vi "GyroServoControl.vi"() -> ()   [LabVIEW 2017]
uses:
  MsgTypeDef.ctl
  <vilib>/WPC Systems Ltd/GECO Driver/Lib/GECOMotion/GECOMotion/_typedefine/Axis Select.ctl
  <vilib>/WPC Systems Ltd/GECO Driver/Lib/GECOMotion/GECOMotion/GECO Motion.lvclass
  <vilib>/WPC Systems Ltd/GECO Driver/Lib/GECOBase/GECO_Driver Class/Motion/_typedefine/GECO_Motion Operation Mode.ctl
  <vilib>/WPC Systems Ltd/GECO Driver/Lib/GECOBase/GECO_Driver Class/GECO_Driver.lvclass
  <vilib>/WPC Systems Ltd/GECO Driver/Lib/GECOBase/GECO_Driver Class/Motion/_typedefine/GECO_ActiveHighLow.ctl
  <vilib>/addons/control/pid/NI_PID_pid.lvlib
  <vilib>/addons/control/pid/pid.llb/PID (DBL).vi
  <vilib>/NI/Modbus Library/API/Wrapper/API Main.lvlib
  GyroDef.ctl
  DataDef.ctl
  <vilib>/WPC Systems Ltd/GECO Driver/Lib/GECOBase/GECO_Driver Class/GECO_SlotName.ctl
  <vilib>/WPC Systems Ltd/GECO Driver/Lib/GECOBase/GECO_Driver Class/Motion/_typedefine/GECO_Stepper Output Configuration.ctl
  <vilib>/NI/Modbus Library/API/Modbus API.lvclass
  <vilib>/Instr/_visa.llb/VISA Configure Serial Port (Instr).vi
  <vilib>/NI/Modbus Library/API/Wrapper/Create TCP Slave.vi
  <vilib>/WPC Systems Ltd/GECO Driver/GECODriver/GECO_Initialize_PC/Initialize VIs/Initialize_GECOUno_4HX.vi
  <vilib>/NI/Modbus Library/API/Slave/Modbus Slave.lvclass
  C:/Program Files (x86)/National Instruments/LabVIEW 2019/vi.lib/NI/Modbus Library/API/Modbus API.lvclass
  Motion Controller Slot.ctl
  Reverse Polarity.ctl
  Forward Polarity.ctl
  Stepper Output Configuration.ctl
  Axis Select.ctl
panel:
  out "error IO 2":errorcluster
  out "error IO":errorcluster
  out "Gyro\nPeriod":u32
  out "Program Period":u32
  out "Axis 3":T1
  out "Axis 2":T1
  out "Axis 1":T1
  in  "ServoButtonControl":T2
  in  "Main Setting Tab":T3(tab)
  in  "TimerON":bool
  in  "Timer(ms)":i32=1
  in  "Serial Port":refnum<visa-resource-name>="COM3"
  in  "TCP slave port":u32=1
  in  "baud rate":u32=115200
  in  "Byte bits":u32=8
  in  "Modbus Address Starting":u32
  in  "Modbus Number of Inputs":u32=10000
  in  "Resource Name":tag="rio://192.168.0.224/RIO0"
  in  "Servo on":bool
  in  "Axis Select":T4
  in  "Stepper Output Configuration":T5=enum."CW/CCW(Two Pulse)"
  in  "Forward Enable?":bool=TRUE
  in  "Reverse Enable?":bool=TRUE
  in  "Motion Operation Mode":T6(ring)=enum."Velocity"
  in  "Forward Polarity":T7
  in  "Reverse Polarity":T8
  in  "Motion Controller Slot":T9
  in  "Target Position (0)":dbl=10000.0
  in  "Acceleration (100000)":u32=300000
  in  "Velocity (10000)":dbl=100000.0
  in  "Deacceleration (100000)":u32=300000
  in  "PID gains setting Tab":enum32{"Axis 1", "Axis 2", "Axis 3"}(tab)
  in  "PID gains":T10={"proportional gain (Kc)"=0.75, "integral time (Ti, min)"=0.01, "derivative time (Td, min)"=0.0} {"derivative time (Td, min)" format="%#_3f"; "integral time (Ti, min)" format="%#_3f"; "proportional gain (Kc)" format="%#_3f"}
  in  "PID gains 2":T10={"proportional gain (Kc)"=0.75, "integral time (Ti, min)"=0.01, "derivative time (Td, min)"=0.0} {"derivative time (Td, min)" format="%#_3f"; "integral time (Ti, min)" format="%#_3f"; "proportional gain (Kc)" format="%#_3f"}
  in  "PID gains 3":T10={"proportional gain (Kc)"=0.75, "integral time (Ti, min)"=0.01, "derivative time (Td, min)"=0.0} {"derivative time (Td, min)" format="%#_3f"; "integral time (Ti, min)" format="%#_3f"; "proportional gain (Kc)" format="%#_3f"}
  in  "ZABStop":bool
  in  "B":i32
  in  "A":i32
  in  "Z":i32=50
  in  "ZAB Start":bool
  in  "Move Setting":T11
  in  "Close":bool
  in  "Connect":bool
  out "實際角度":cluster{"A":dbl, "B":dbl}={"A"=-3.299667554384925, "B"=3.520332445615068}
  out "register values":dbl[](array[numeric])
  out "實際角度Chart":cluster{"X":dbl, "Y":dbl}(graph)={"X"=-3.299667554384925, "Y"=3.520332445615068} caption="Waveform Chart - dark"
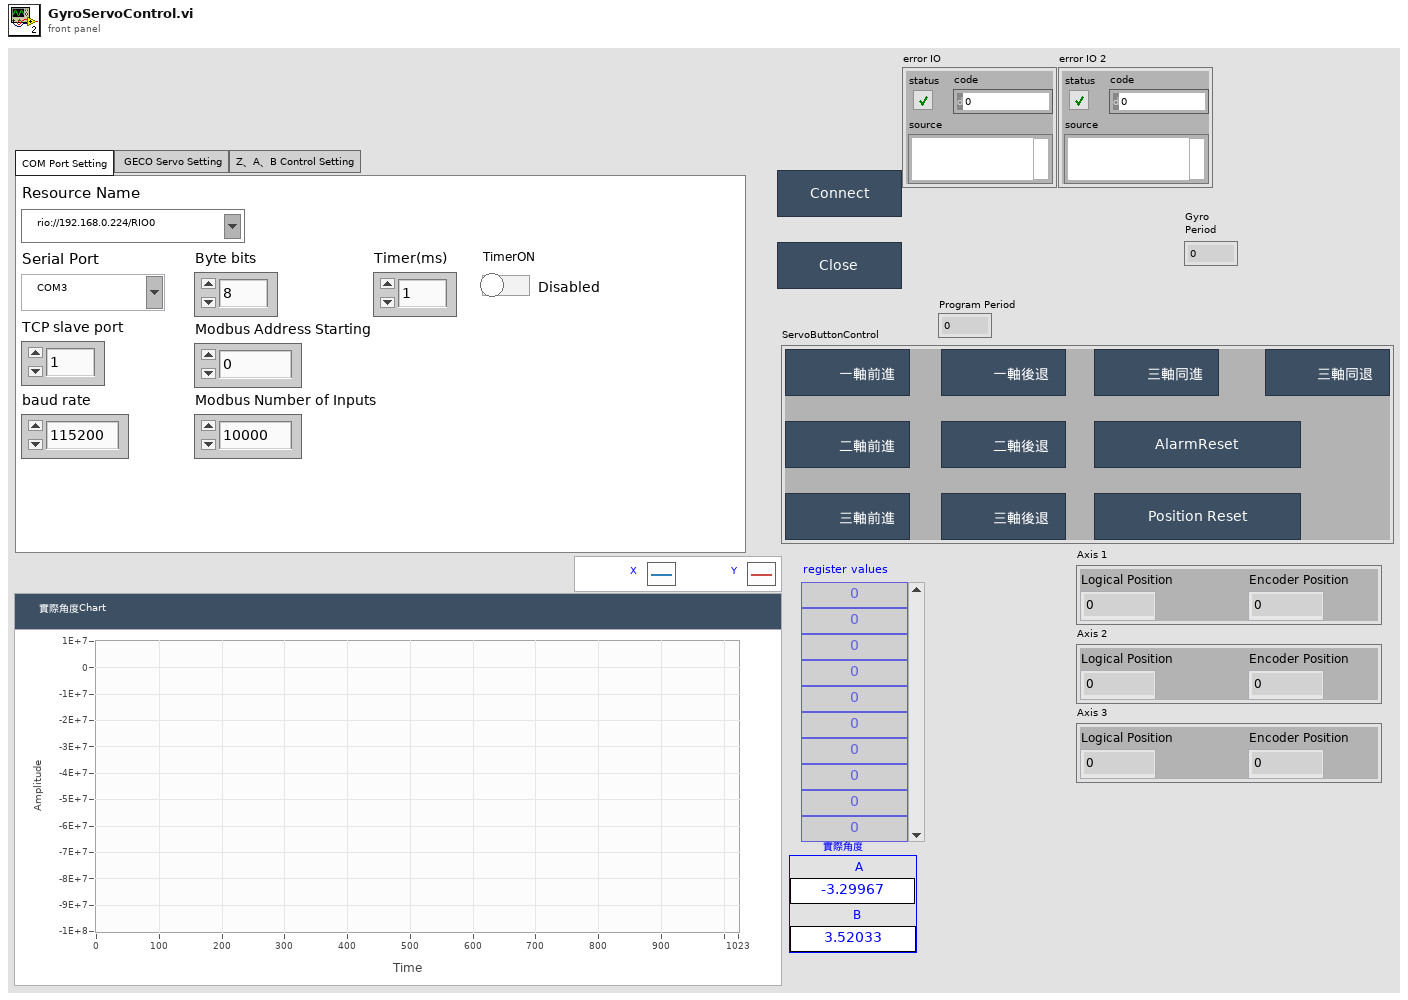
[diagram p1: front panel]
types:
  T1 = cluster{"Encoder Position":i32, "Logical Position":i32}
  T2 = cluster{"三軸同退":bool, "三軸同進":bool, "三軸後退":bool, "三軸前進":bool, "二軸後退":bool, "二軸前進":bool, "一軸後退":bool, "一軸前進":bool, "Reset Encoder Position":bool, "AlarmReset":bool}
  T3 = enum32{"COM Port Setting", " GECO Servo Setting", "Z、A、B Control Setting"}
  T4 = typedef "Axis Select.ctl" = enum16{"Axis 1", "Axis 2", "Axis 3", "Axis 4"}
  T5 = typedef "Stepper Output Configuration.ctl" = enum16{"Step/Dir(One Pulse)", "CW/CCW(Two Pulse)"}
  T6 = enum16{"Absolute Position", "Relative Position", "Velocity"}
  T7 = typedef "Forward Polarity.ctl" = enum16{"Active High", "Active Low"}
  T8 = typedef "Reverse Polarity.ctl" = enum16{"Active High", "Active Low"}
  T9 = typedef "Motion Controller Slot.ctl" = enum16{"C1", "C2", "C3", "C4"}
  T10 = cluster{"proportional gain (Kc)":dbl, "integral time (Ti, min)":dbl, "derivative time (Td, min)":dbl}
  T11 = typedef "軌跡設定.ctl" = u16
  T12 = typedef "MsgTypeDef.ctl" = cluster{"CMD":string, "DATA":variant}
  T13 = typedef "GyroDef.ctl" = cluster{"Byte bits":u16, "baud rate":u32, "實際角度":cluster{"A":dbl, "B":dbl}, "COM Port":refnum<visa-resource-name>, "Save Path":refnum<file>}
  T14 = typedef "DataDef.ctl" = cluster{"address starting":u16, "狀態":enum16{"初始化", "讀取", "寫入", "停止"}, "理想角度":cluster{"A":dbl, "B":dbl}, "register values":i16[], "Modbus COM":refnum<class "Modbus API.lvclass">, "TCP slave port":u16, " baud rate":u32, "Byte bits":u16, "ServoButtonControl":cluster{"三軸同退":bool, "三軸同進":bool, "三軸後退":bool, "三軸前進":bool, "二軸後退":bool, "二軸前進":bool, "一軸後退":bool, "一軸前進":bool}, "Serial Number":string, "GECO_Driver out":refnum<class "GECO_Driver.lvclass">, "number of inputs":u16, "ServoSetting":cluster{"Axis Select":T15, "Stepper Output Configuration":T16, "Motion Operation Mode":T17, "Motion Controller Slot":T18, "Singel Axis Move Paramters":cluster{"Motion Operation Mode":T17, "Target Position (0)":i32, "Velocity (10000)":i32, "Acceleration (100000)":u32, "Deacceleration (100000)":u32}, "Reverse":cluster{"Reverse Enable":bool, "Reverse Polarity":T19}, "Forward":cluster{"Forward Enable":bool, "Forward Polarity":T19}}, "GECO Motion out":refnum<class "GECO Motion.lvclass">, "Servo on":bool, "Axis 1 Position":cluster{"Encoder Position":i32, "Logical Position":i32}, "Axis 2 Position":cluster{"Encoder Position":i32, "Logical Position":i32}, "Axis 3 Position":cluster{"Encoder Position":i32, "Logical Position":i32}, "PIDSetting":cluster{"Z":i32, "A":i32, "B":i32, "Move Setting":T20, "Axis Pulse":dbl, "Axis Length":dbl, "PID gains ":cluster{"proportional gain (Kc)":dbl, "integral time (Ti, min)":dbl, "derivative time (Td, min)":dbl}}, "resource name":tag, "Save Path":refnum<file>}
  T15 = typedef "GECO Motion.lvclass/Axis Select.ctl" = enum16{"Axis 1", "Axis 2", "Axis 3", "Axis 4"}
  T16 = typedef "GECO_Driver.lvclass/GECO_Stepper Output Configuration.ctl" = enum16{"Step/Dir(One Pulse)", "CW/CCW(Two Pulse)"}
  T17 = typedef "GECO_Driver.lvclass/GECO_Motion Operation Mode.ctl" = enum16{"Absolute Position", "Relative Position", "Velocity"}
  T18 = typedef "GECO_Driver.lvclass/GECO_SlotName.ctl" = enum16{"C1", "C2", "C3", "C4"}
  T19 = typedef "GECO_Driver.lvclass/GECO_ActiveHighLow.ctl" = enum16{"Active High", "Active Low"}
  T20 = typedef "­y¸ñ.ctl" = u16
  T21 = cluster{"Motion Operation Mode":T17, "Target Position (0)":i32, "Velocity (10000)":i32, "Acceleration (100000)":u32, "Deacceleration (100000)":u32}
  T22 = cluster{"Forward Enable":bool, "Forward Polarity":T19}
  T23 = cluster{"Reverse Enable":bool, "Reverse Polarity":T19}
  T24 = cluster{"三軸同退":bool, "三軸同進":bool, "三軸後退":bool, "三軸前進":bool, "二軸後退":bool, "二軸前進":bool, "一軸後退":bool, "一軸前進":bool, "Reset Encoder Position":bool, "AlarmReset":bool}[]
  T25 = enum16{"open", "replace", "create", "open or create", "replace or create", "replace or create with confirmation"}
  T26 = cluster{"Logical Position":i32, "Encoder Position":i32}
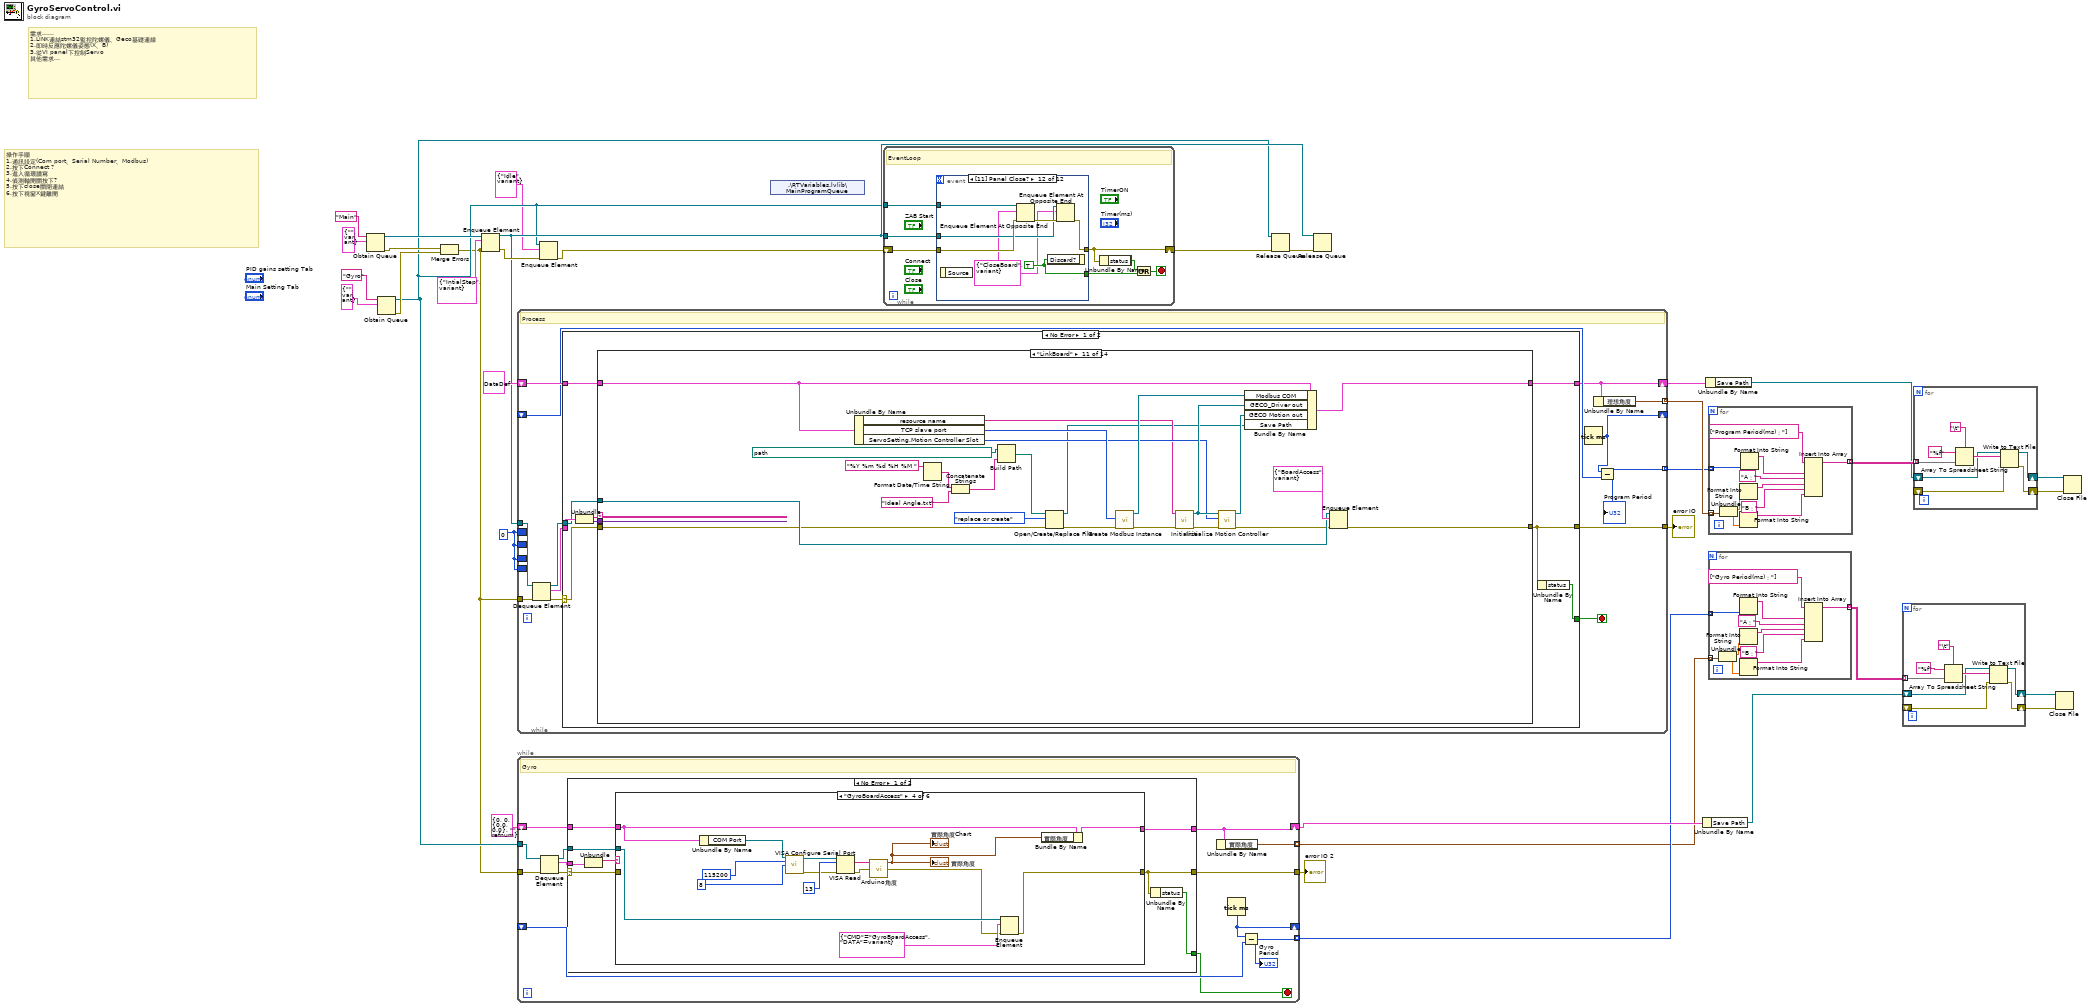
[diagram p0: block diagram]
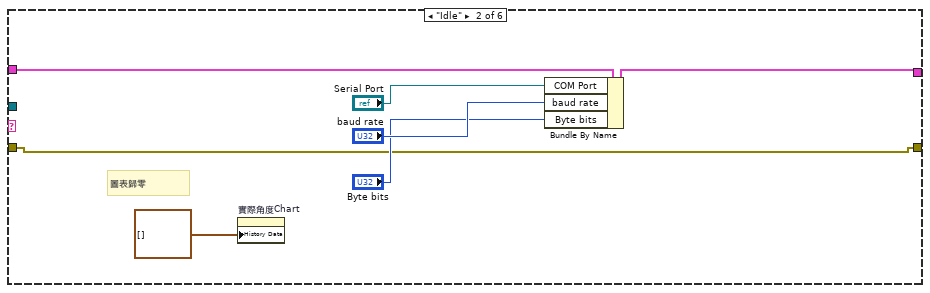
[diagram p3: hidden frame]
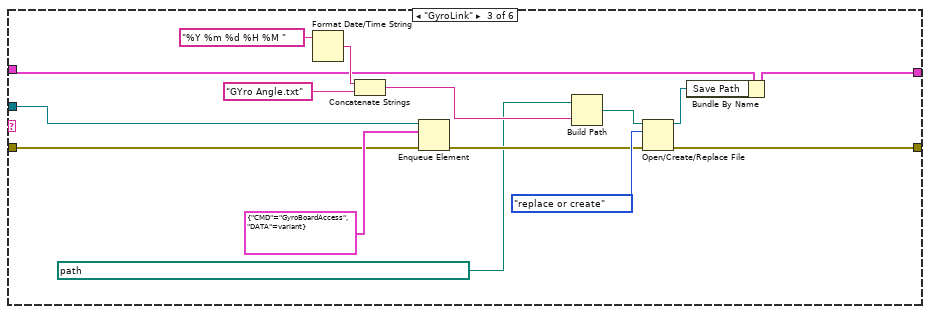
[diagram p4: hidden frame]
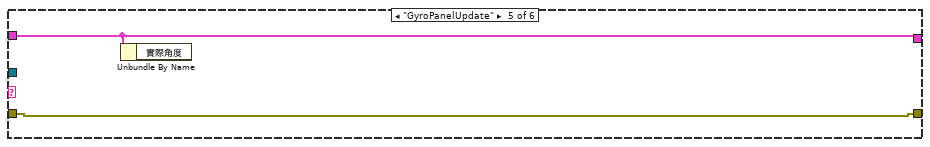
[diagram p5: hidden frame]
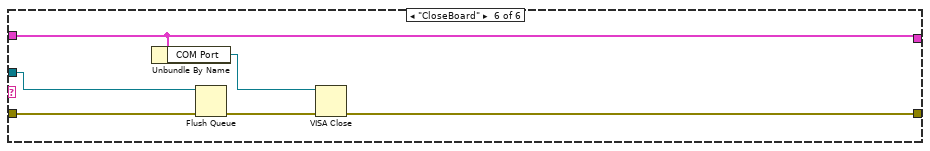
[diagram p6: hidden frame]
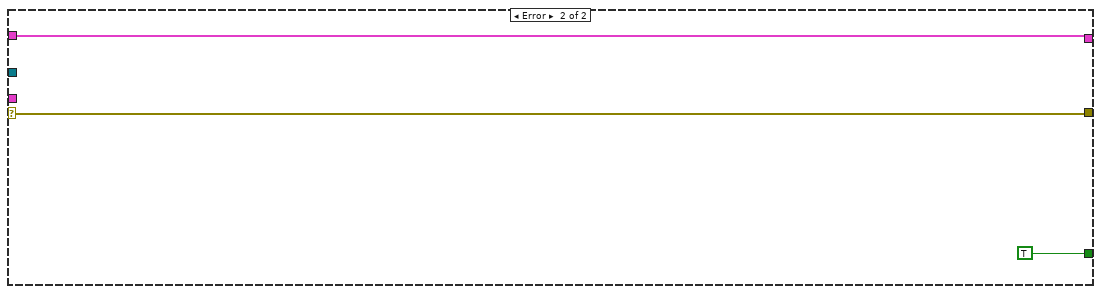
[diagram p7: hidden frame]
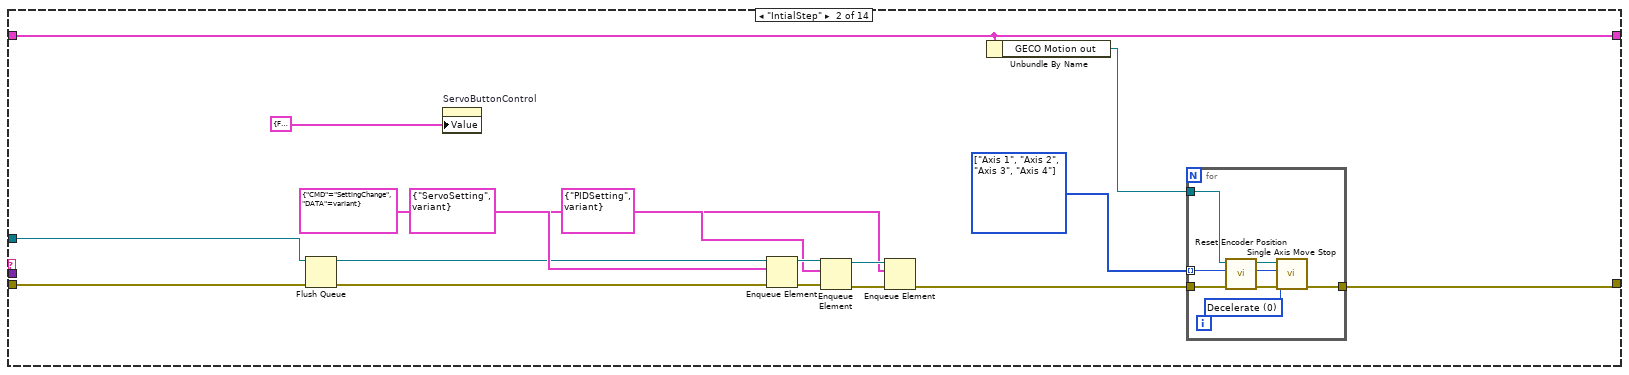
[diagram p9: hidden frame]
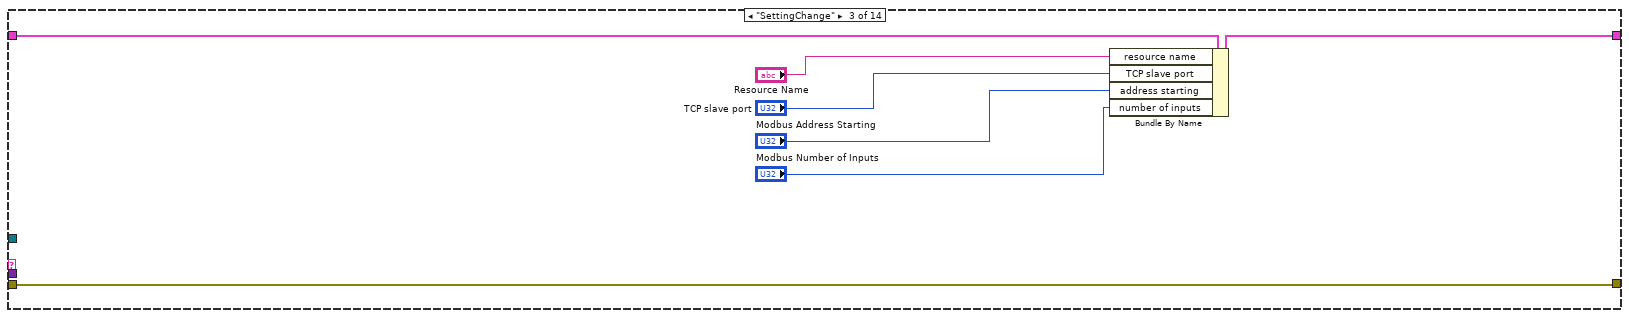
[diagram p10: hidden frame]
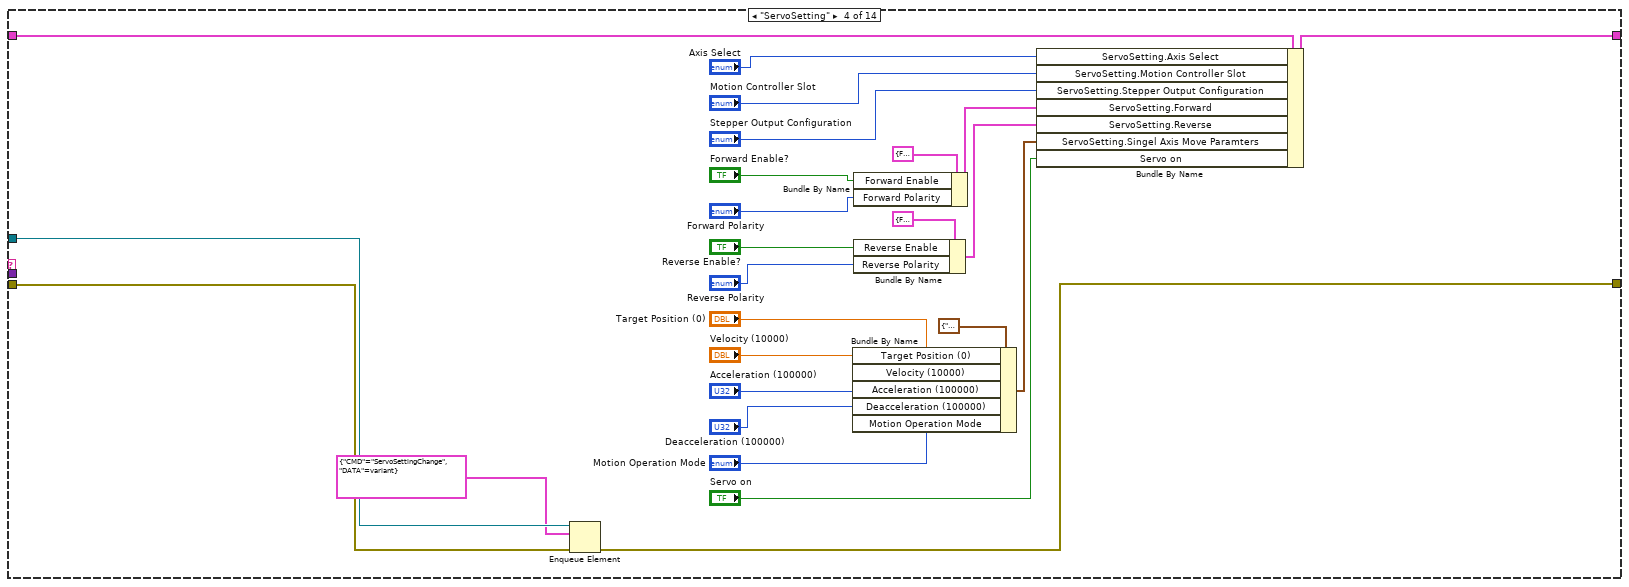
[diagram p11: hidden frame]
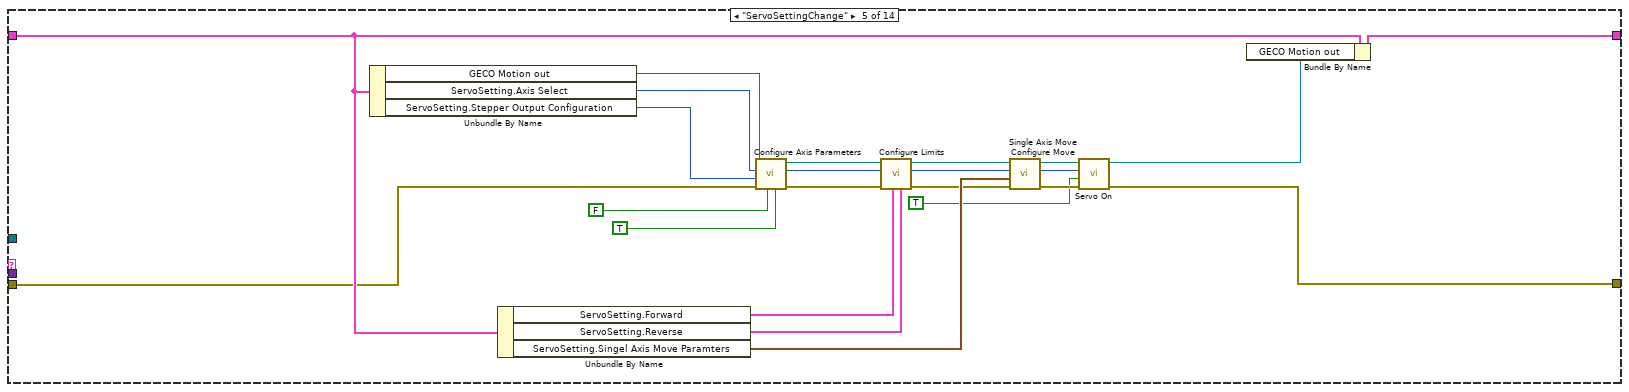
[diagram p12: hidden frame]
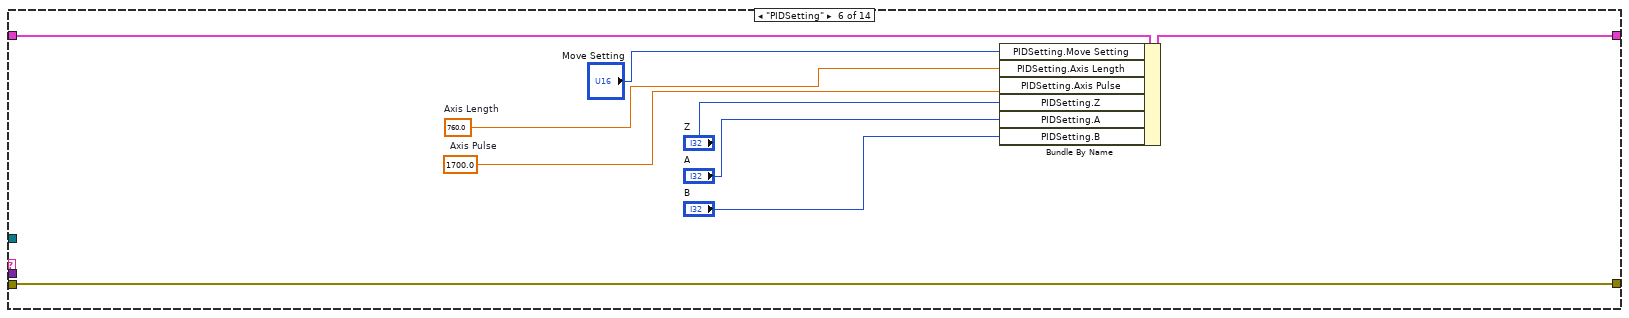
[diagram p13: hidden frame]
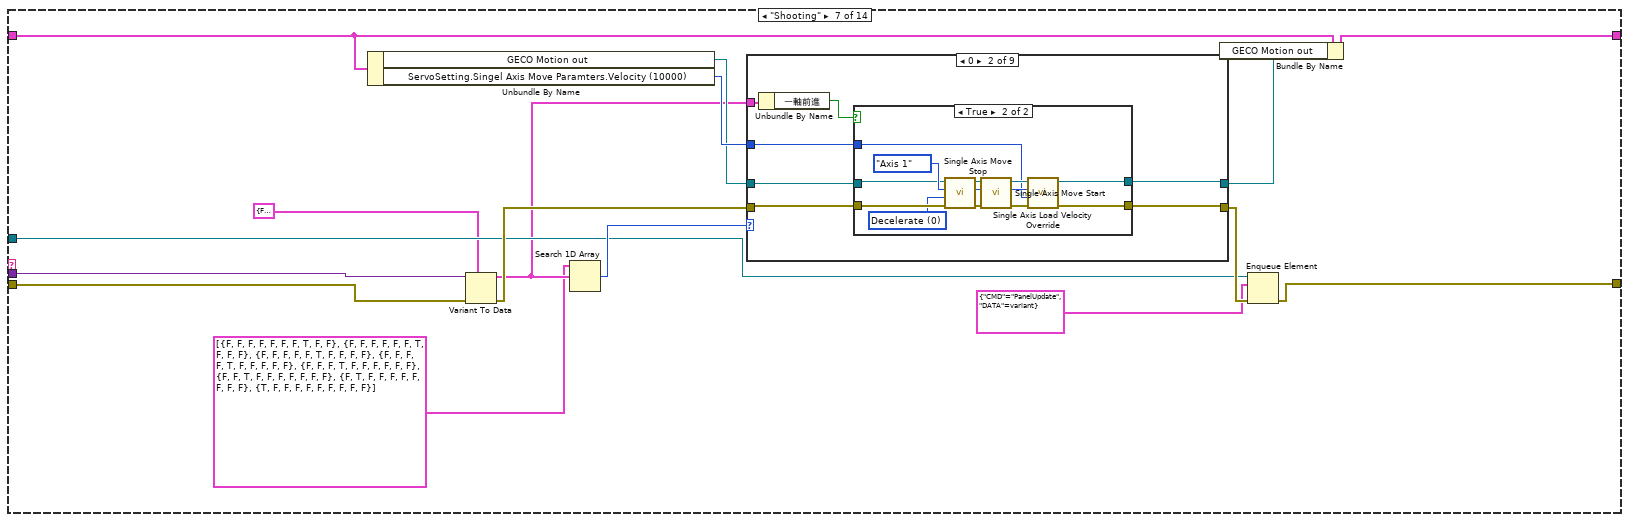
[diagram p14: hidden frame]
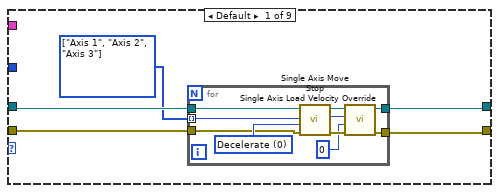
[diagram p15: hidden frame]
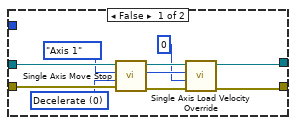
[diagram p16: hidden frame]
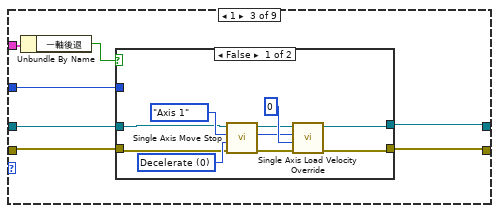
[diagram p17: hidden frame]
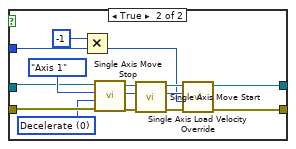
[diagram p18: hidden frame]
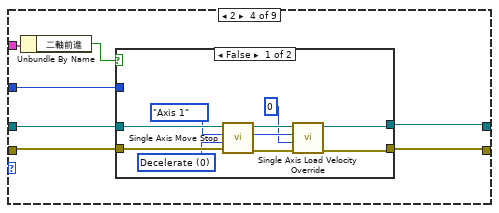
[diagram p19: hidden frame]
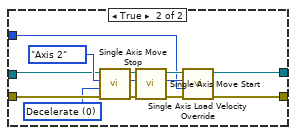
[diagram p20: hidden frame]
diagram:
  w17 = 0
  # "操作手順\n1.通訊設定(Com port、Serial Number、Modbus)\n2.按下Connect ?\n3.進入循環讀寫\n4.偵測軸開關按下?\n5.按下close關閉連結\n6.按下視窗X鍵離開"
  # "需求......\n1.LINK連結stm32監控陀螺儀、Geco基礎連線\n2.即時反應陀螺儀姿態(X、B)\n3.從VI panel下控制Servo\n其他需求..."
  n1 = Obtain Queue(name (unnamed)="Main", element data type=T12 {"CMD"="", "DATA"=variant}) -> (queue out=w31:refnum<queue>, error out=w26:errorcluster)  [unwired: 3 in, 1 out]
  n2 = Obtain Queue(name (unnamed)="Gyro", element data type=T12 {"CMD"="", "DATA"=variant}) -> (queue out=w21:refnum<queue>, error out=w27:errorcluster)  [unwired: 3 in, 1 out]
  n3 = Merge Errors(w26, w27) -> (w19:errorcluster)
  n4 = Enqueue Element(queue=w31, element=T12 {"CMD"="IntialStep", "DATA"=variant}, error in (no error)=w19) -> (queue out=w22:refnum<queue>, error out=w24:errorcluster)  [unwired: 1 in, 1 out]
  n5 = while {
    tunnel: w22 -> [w48]
    shift-right: [w39] -> w13
    shift-left: T14 {"address starting"=0, "狀態"=enum."初始化", "理想角度"={"A"=0.0, "B"=0.0}, "register values"=[], "Modbus COM"=refnum, "TCP slave port"=1, " baud rate"=0, "Byte bits"=0, "ServoButtonControl"={"三軸同退"=FALSE, "三軸同進"=FALSE, "三軸後退"=FALSE, "三軸前進"=FALSE, "二軸後退"=FALSE, "二軸前進"=FALSE, "一軸後退"=FALSE, "一軸前進"=FALSE}, "Serial Number"="", "GECO_Driver out"=refnum, "number of inputs"=0, "ServoSetting"={"Axis Select"=enum."Axis 1", "Stepper Output Configuration"=enum."Step/Dir(One Pulse)", "Motion Operation Mode"=enum."Absolute Position", "Motion Controller Slot"=enum."C1", "Singel Axis Move Paramters"={"Motion Operation Mode"=enum."Velocity", "Target Position (0)"=10000, "Velocity (10000)"=1, "Acceleration (100000)"=100000, "Deacceleration (100000)"=1}, "Reverse"={"Reverse Enable"=FALSE, "Reverse Polarity"=enum."Active Low"}, "Forward"={"Forward Enable"=FALSE, "Forward Polarity"=enum."Active Low"}}, "GECO Motion out"=refnum, "Servo on"=FALSE, "Axis 1 Position"={"Encoder Position"=0, "Logical Position"=0}, "Axis 2 Position"={"Encoder Position"=0, "Logical Position"=0}, "Axis 3 Position"={"Encoder Position"=0, "Logical Position"=0}, "PIDSetting"={"Z"=10000, "A"=10000, "B"=10000, "Move Setting"=1, "Axis Pulse"=10000.0, "Axis Length"=10000.0, "PID gains "={"proportional gain (Kc)"=1.0, "integral time (Ti, min)"=0.01, "derivative time (Td, min)"=0.0}}, "resource name"="", "Save Path"=refnum} -> [w44]
    tunnel: w19 -> [w42]
    shift-right: [w41] -> _
    shift-left: _ -> [w40]
    border: w17 -> [_]
    border: w17 -> [_]
    border: w17 -> [_]
    border: w17 -> [_]
    tunnel: [w38] -> w16 mode=indexing
    tunnel: [w37] -> w15 mode=indexing
    tunnel: [w36] -> w2
    stop <- w45 stop-if-true
    # "Process"
    n6 = Dequeue Element(queue=w48, error in (no error)=w42) -> (queue out=w43:refnum<queue>, element=w46:T12, error out=w47:errorcluster)  [unwired: 1 in, 1 out]
    n7 = case shown="No Error" w47 {
      selector: w47 -> [w53 w718]
      tunnel: w46 -> [w57 _]
      tunnel: [w50 TRUE] -> w45
      tunnel: [w55 w719] -> w39
      tunnel: w44 -> [w54 w719]
      tunnel: w43 -> [w52 _]
      tunnel: [w49 w718] -> w36
      frame No Error {
        n8 = Unbundle(w57) -> ("CMD"=w56:string, "DATA"=w51:variant)
        n9 = case shown="\"LinkBoard\"" w56 {
          tunnel: [w59 w60 w90 w115 w139 w147 w162 w453 w607 w623 w659 w673 w695 w709] -> w55
          tunnel: w54 -> [w59 w60 w91 w116 w138 w148 w156 w455 w610 w626 w660 w674 w697 w709]
          tunnel: w53 -> [w58 w64 w87 w94 w131 w140 w164 w445 w609 w625 w639 w667 w699 w706]
          tunnel: [w58 w71 w87 w92 w125 w140 w153 w454 w605 w621 w656 w664 w698 w708] -> w49
          tunnel: w52 -> [_ w65 _ w95 _ _ w154 w451 _ _ w654 w668 _ w707]
          tunnel: w51 -> [_ _ _ _ _ _ w163 _ _ _ _ _ _ _]
          frame Default {
          }
          frame "IntialStep" {
            w69 = T15[] [enum."Axis 1", enum."Axis 2", enum."Axis 3", enum."Axis 4"] items=["Axis 1", "Axis 2", "Axis 3", "Axis 4"]
            n10 = Flush Queue(queue=w65, error in (no error)=w64) -> (queue out=w63:refnum<queue>, error out=w62:errorcluster)  [unwired: 1 out]
            n11 = property on="ServoButtonControl" class="Clust"("Value"=T2 {"三軸同退"=FALSE, "三軸同進"=FALSE, "三軸後退"=FALSE, "三軸前進"=FALSE, "二軸後退"=FALSE, "二軸前進"=FALSE, "一軸後退"=FALSE, "一軸前進"=FALSE, "Reset Encoder Position"=FALSE, "AlarmReset"=FALSE} ("ServoButtonControl")) -> ()  [unwired: 2 in, 2 out]
            n12 = Enqueue Element(queue=w63, element=T12 {"CMD"="SettingChange", "DATA"=variant}, error in (no error)=w62) -> (queue out=w74:refnum<queue>, error out=w75:errorcluster)  [unwired: 1 in, 1 out]
            n13 = Enqueue Element(queue=w74, element=T12 {"CMD"="ServoSetting", "DATA"=variant}, error in (no error)=w75) -> (queue out=w68:refnum<queue>, error out=w67:errorcluster)  [unwired: 1 in, 1 out]
            n14 = Enqueue Element(queue=w68, element=T12 {"CMD"="PIDSetting", "DATA"=variant}, error in (no error)=w67) -> (error out=w61:errorcluster)  [unwired: 1 in, 2 out]
            n15 = Unbundle By Name(w60) -> ("GECO Motion out"=w70:refnum<class "GECO Motion.lvclass">)
            n16 = for {
              tunnel: w61 -> [w84]
              tunnel: [w78] -> w71
              tunnel: w70 -> [w83]
              tunnel: w69 -> [w82] mode=indexing
              w77 = u16 0 items=["Decelerate", "Halt"] ("Motion Stop Type")
              n17 = call <vilib>:"Reset Encoder Position.vi"("error in (no error)"=w84, "Axis Select"=w82, "GECO Motion in"=w83) -> ("error out"=w81:errorcluster, "Axis Select out"=w80:T15, "GECO Motion out"=w79:refnum<class "GECO Motion.lvclass">)  [unwired: 6 in]
              n18 = call <vilib>:"Single Axis Move Stop.vi"("error in (no error)"=w81, "Motion Stop Type"=w77, "Axis Select"=w80, "GECO Motion in"=w79) -> ("error out"=w78:errorcluster)  [unwired: 5 in, 2 out]
            }
          }
          frame "SettingChange" {
            n19 = Bundle By Name(cluster=w91, "resource name"="Resource Name", "TCP slave port"="TCP slave port", "address starting"="Modbus Address Starting", "number of inputs"="Modbus Number of Inputs") -> (w90:T14)
          }
          frame "ServoSetting" {
            n20 = Enqueue Element(queue=w95, element=T12 {"CMD"="ServoSettingChange", "DATA"=variant}, error in (no error)=w94) -> (error out=w92:errorcluster)  [unwired: 1 in, 2 out]
            n21 = Bundle By Name(cluster=T21 {"Motion Operation Mode"=enum."Absolute Position", "Target Position (0)"=0, "Velocity (10000)"=10000, "Acceleration (100000)"=100000, "Deacceleration (100000)"=100000} ("Singel Axis Move Paramters"), "Target Position (0)"="Target Position (0)", "Velocity (10000)"="Velocity (10000)", "Acceleration (100000)"="Acceleration (100000)", "Deacceleration (100000)"="Deacceleration (100000)", "Motion Operation Mode"="Motion Operation Mode") -> (w97:T21)
            n22 = Bundle By Name(cluster=T22 {"Forward Enable"=FALSE, "Forward Polarity"=enum."Active Low"} ("Forward"), "Forward Enable"="Forward Enable?", "Forward Polarity"="Forward Polarity") -> (w99:T22)
            n23 = Bundle By Name(cluster=T23 {"Reverse Enable"=FALSE, "Reverse Polarity"=enum."Active Low"} ("Reverse"), "Reverse Enable"="Reverse Enable?", "Reverse Polarity"="Reverse Polarity") -> (w98:T23)
            n24 = Bundle By Name(cluster=w116, "ServoSetting.Axis Select"="Axis Select", "ServoSetting.Motion Controller Slot"="Motion Controller Slot", "ServoSetting.Stepper Output Configuration"="Stepper Output Configuration", "ServoSetting.Forward"=w99, "ServoSetting.Reverse"=w98, "ServoSetting.Singel Axis Move Paramters"=w97, "Servo on"="Servo on") -> (w115:T14)
          }
          frame "ServoSettingChange" {
            n25 = Unbundle By Name(w138) -> ("GECO Motion out"=w132:refnum<class "GECO Motion.lvclass">, "ServoSetting.Axis Select"=w136:T15, "ServoSetting.Stepper Output Configuration"=w135:T16)
            n26 = Unbundle By Name(w138) -> ("ServoSetting.Forward"=w118:T22, "ServoSetting.Reverse"=w117:T23, "ServoSetting.Singel Axis Move Paramters"=w137:T21)
            n27 = call <vilib>:"Configure Axis Parameters.vi"("Reverse Encoder Direction?"=TRUE, "Reverse Axis Direction?"=FALSE, "error in (no error)"=w131, "Stepper Output Configuration"=w135, "Axis Select"=w136, "GECO Motion in"=w132) -> ("error out"=w122:errorcluster, "Axis Select out"=w124:T15, "GECO Motion out"=w123:refnum<class "GECO Motion.lvclass">)  [unwired: 3 in]
            n28 = call <vilib>:"Configure Limits.vi"("Reverse"=w117, "Forward"=w118, "error in (no error)"=w122, "Axis Select"=w124, "GECO Motion in"=w123) -> ("error out"=w119:errorcluster, "Axis Select out"=w120:T15, "GECO Motion out"=w121:refnum<class "GECO Motion.lvclass">)  [unwired: 4 in]
            n29 = call <vilib>:"Single Axis Move Configure Move.vi"("error in (no error)"=w119, "Singel Axis Move Paramters"=w137, "Axis Select"=w120, "GECO Motion in"=w121) -> ("error out"=w128:errorcluster, "Axis Select out"=w129:T15, "GECO Motion out"=w130:refnum<class "GECO Motion.lvclass">)  [unwired: 5 in]
            n30 = call <vilib>:"Servo On.vi"("error in (no error)"=w128, "Servo On"=TRUE, "Axis Select"=w129, "GECO Motion in"=w130) -> ("error out"=w125:errorcluster, "GECO Motion out"=w126:refnum<class "GECO Motion.lvclass">)  [unwired: 5 in, 1 out]
            n31 = Bundle By Name(cluster=w138, "GECO Motion out"=w126) -> (w139:T14)
          }
          frame "PIDSetting" {
            w144 = 1700.0  # Axis Pulse
            w145 = 760.0  # Axis Length
            n32 = Bundle By Name(cluster=w148, "PIDSetting.Move Setting"="Move Setting", "PIDSetting.Axis Length"=w145, "PIDSetting.Axis Pulse"=w144, "PIDSetting.Z"="Z", "PIDSetting.A"="A", "PIDSetting.B"="B") -> (w147:T14)
          }
          frame "Shooting" {
            n33 = Unbundle By Name(w156) -> ("GECO Motion out"=w158:refnum<class "GECO Motion.lvclass">, "ServoSetting.Singel Axis Move Paramters.Velocity (10000)"=w159:i32)
            n34 = Variant To Data(error in=w164, type=T2 {"三軸同退"=FALSE, "三軸同進"=FALSE, "三軸後退"=FALSE, "三軸前進"=FALSE, "二軸後退"=FALSE, "二軸前進"=FALSE, "一軸後退"=FALSE, "一軸前進"=FALSE, "Reset Encoder Position"=FALSE, "AlarmReset"=FALSE} ("ServoButtonControl"), Variant=w163) -> (data=w151:T2, error out=w160:errorcluster)
            n35 = Search 1D Array(1D array=T24 [{"三軸同退"=FALSE, "三軸同進"=FALSE, "三軸後退"=FALSE, "三軸前進"=FALSE, "二軸後退"=FALSE, "二軸前進"=FALSE, "一軸後退"=FALSE, "一軸前進"=TRUE, "Reset Encoder Position"=FALSE, "AlarmReset"=FALSE}, {"三軸同退"=FALSE, "三軸同進"=FALSE, "三軸後退"=FALSE, "三軸前進"=FALSE, "二軸後退"=FALSE, "二軸前進"=FALSE, "一軸後退"=TRUE, "一軸前進"=FALSE, "Reset Encoder Position"=FALSE, "AlarmReset"=FALSE}, {"三軸同退"=FALSE, "三軸同進"=FALSE, "三軸後退"=FALSE, "三軸前進"=FALSE, "二軸後退"=FALSE, "二軸前進"=TRUE, "一軸後退"=FALSE, "一軸前進"=FALSE, "Reset Encoder Position"=FALSE, "AlarmReset"=FALSE}, {"三軸同退"=FALSE, "三軸同進"=FALSE, "三軸後退"=FALSE, "三軸前進"=FALSE, "二軸後退"=TRUE, "二軸前進"=FALSE, "一軸後退"=FALSE, "一軸前進"=FALSE, "Reset Encoder Position"=FALSE, "AlarmReset"=FALSE}, {"三軸同退"=FALSE, "三軸同進"=FALSE, "三軸後退"=FALSE, "三軸前進"=TRUE, "二軸後退"=FALSE, "二軸前進"=FALSE, "一軸後退"=FALSE, "一軸前進"=FALSE, "Reset Encoder Position"=FALSE, "AlarmReset"=FALSE}, {"三軸同退"=FALSE, "三軸同進"=FALSE, "三軸後退"=TRUE, "三軸前進"=FALSE, "二軸後退"=FALSE, "二軸前進"=FALSE, "一軸後退"=FALSE, "一軸前進"=FALSE, "Reset Encoder Position"=FALSE, "AlarmReset"=FALSE}, {"三軸同退"=FALSE, "三軸同進"=TRUE, "三軸後退"=FALSE, "三軸前進"=FALSE, "二軸後退"=FALSE, "二軸前進"=FALSE, "一軸後退"=FALSE, "一軸前進"=FALSE, "Reset Encoder Position"=FALSE, "AlarmReset"=FALSE}, {"三軸同退"=TRUE, "三軸同進"=FALSE, "三軸後退"=FALSE, "三軸前進"=FALSE, "二軸後退"=FALSE, "二軸前進"=FALSE, "一軸後退"=FALSE, "一軸前進"=FALSE, "Reset Encoder Position"=FALSE, "AlarmReset"=FALSE}], element=w151) -> (index of element=w161:i32)  [unwired: 1 in]
            n36 = case shown="0" w161 {
              tunnel: w160 -> [w168 w185 w215 w247 w277 w309 w339 w371 w408]
              tunnel: w159 -> [_ w184 w214 w246 w276 w308 w338 w370 w407]
              tunnel: w158 -> [w169 w186 w216 w248 w278 w310 w340 w372 w409]
              tunnel: [w166 w183 w213 w245 w275 w307 w337 w369 w406] -> w157
              tunnel: [w165 w182 w212 w244 w274 w306 w336 w368 w405] -> w155
              tunnel: w151 -> [_ w181 w211 w243 w273 w305 w335 w367 w404]
              frame Default {
                w167 = T15[] [enum."Axis 1", enum."Axis 2", enum."Axis 3"] items=["Axis 1", "Axis 2", "Axis 3", "Axis 4"] ("Start Axes Select")
                n37 = for {
                  tunnel: w168 -> [w178]
                  tunnel: w169 -> [w177]
                  tunnel: w167 -> [w176] mode=indexing
                  tunnel: [w171] -> w166
                  tunnel: [w172] -> w165
                  w179 = u16 0 items=["Decelerate", "Halt"] ("Motion Stop Type")
                  n38 = call <vilib>:"Single Axis Move Stop.vi"("error in (no error)"=w178, "Motion Stop Type"=w179, "Axis Select"=w176, "GECO Motion in"=w177) -> ("error out"=w174:errorcluster, "Axis Select out"=w173:T15, "GECO Motion out"=w175:refnum<class "GECO Motion.lvclass">)  [unwired: 5 in]
                  n39 = call <vilib>:"Single Axis Load Velocity Override.vi"("error in (no error)"=w174, "Override Velosity Value"=0, "Axis Select"=w173, "GECO Motion in"=w175) -> ("error out"=w172:errorcluster, "GECO Motion out"=w171:refnum<class "GECO Motion.lvclass">)  [unwired: 5 in, 1 out]
                }
              }
              frame 0 {
                n40 = Unbundle By Name(w181) -> ("一軸前進"=w180:bool)
                n41 = case shown="True" w180 {
                  tunnel: w186 -> [w196 w202]
                  tunnel: w185 -> [w195 w201]
                  tunnel: w184 -> [_ w206]
                  tunnel: [w187 w205] -> w183
                  tunnel: [w188 w204] -> w182
                  frame False {
                    w194 = u16 0 items=["Decelerate", "Halt"] ("Motion Stop Type")
                    n42 = call <vilib>:"Single Axis Move Stop.vi"("error in (no error)"=w195, "Motion Stop Type"=w194, "Axis Select"=Axis_Select."Axis 1", "GECO Motion in"=w196) -> ("error out"=w191:errorcluster, "Axis Select out"=w190:T15, "GECO Motion out"=w192:refnum<class "GECO Motion.lvclass">)  [unwired: 5 in]
                    n43 = call <vilib>:"Single Axis Load Velocity Override.vi"("error in (no error)"=w191, "Override Velosity Value"=0, "Axis Select"=w190, "GECO Motion in"=w192) -> ("error out"=w188:errorcluster, "GECO Motion out"=w187:refnum<class "GECO Motion.lvclass">)  [unwired: 5 in, 1 out]
                  }
                  frame True {
                    w200 = u16 0 items=["Decelerate", "Halt"] ("Motion Stop Type")
                    n44 = call <vilib>:"Single Axis Move Stop.vi"("error in (no error)"=w201, "Motion Stop Type"=w200, "Axis Select"=Axis_Select."Axis 1", "GECO Motion in"=w202) -> ("error out"=w198:errorcluster, "Axis Select out"=w197:T15, "GECO Motion out"=w199:refnum<class "GECO Motion.lvclass">)  [unwired: 5 in]
                    n45 = call <vilib>:"Single Axis Move Start.vi"("error in (no error)"=w198, "Axis Select"=w197, "GECO Motion in"=w199) -> ("error out"=w208:errorcluster, "Axis Select out"=w207:T15, "GECO Motion out"=w209:refnum<class "GECO Motion.lvclass">)  [unwired: 6 in]
                    n46 = call <vilib>:"Single Axis Load Velocity Override.vi"("error in (no error)"=w208, "Override Velosity Value"=w206, "Axis Select"=w207, "GECO Motion in"=w209) -> ("error out"=w204:errorcluster, "GECO Motion out"=w205:refnum<class "GECO Motion.lvclass">)  [unwired: 5 in, 1 out]
                  }
                }
              }
              frame 1 {
                n47 = Unbundle By Name(w211) -> ("一軸後退"=w210:bool)
                n48 = case shown="False" w210 {
                  tunnel: w216 -> [w222 w230]
                  tunnel: w215 -> [w220 w229]
                  tunnel: w214 -> [_ w238]
                  tunnel: [w224 w237] -> w213
                  tunnel: [w225 w236] -> w212
                  frame False {
                    w221 = u16 0 items=["Decelerate", "Halt"] ("Motion Stop Type")
                    n49 = call <vilib>:"Single Axis Move Stop.vi"("error in (no error)"=w220, "Motion Stop Type"=w221, "Axis Select"=Axis_Select."Axis 1", "GECO Motion in"=w222) -> ("error out"=w218:errorcluster, "Axis Select out"=w217:T15, "GECO Motion out"=w219:refnum<class "GECO Motion.lvclass">)  [unwired: 5 in]
                    n50 = call <vilib>:"Single Axis Load Velocity Override.vi"("error in (no error)"=w218, "Override Velosity Value"=0, "Axis Select"=w217, "GECO Motion in"=w219) -> ("error out"=w225:errorcluster, "GECO Motion out"=w224:refnum<class "GECO Motion.lvclass">)  [unwired: 5 in, 1 out]
                  }
                  frame True {
                    w228 = u16 0 items=["Decelerate", "Halt"] ("Motion Stop Type")
                    n51 = Multiply(x=-1, y=w238) -> (x*y=w235:i32)
                    n52 = call <vilib>:"Single Axis Move Stop.vi"("error in (no error)"=w229, "Motion Stop Type"=w228, "Axis Select"=Axis_Select."Axis 1", "GECO Motion in"=w230) -> ("error out"=w232:errorcluster, "Axis Select out"=w227:T15, "GECO Motion out"=w233:refnum<class "GECO Motion.lvclass">)  [unwired: 5 in]
                    n53 = call <vilib>:"Single Axis Move Start.vi"("error in (no error)"=w232, "Axis Select"=w227, "GECO Motion in"=w233) -> ("error out"=w240:errorcluster, "Axis Select out"=w239:T15, "GECO Motion out"=w241:refnum<class "GECO Motion.lvclass">)  [unwired: 6 in]
                    n54 = call <vilib>:"Single Axis Load Velocity Override.vi"("error in (no error)"=w240, "Override Velosity Value"=w235, "Axis Select"=w239, "GECO Motion in"=w241) -> ("error out"=w236:errorcluster, "GECO Motion out"=w237:refnum<class "GECO Motion.lvclass">)  [unwired: 5 in, 1 out]
                  }
                }
              }
              frame 2 {
                n55 = Unbundle By Name(w243) -> ("二軸前進"=w242:bool)
                n56 = case shown="False" w242 {
                  tunnel: w248 -> [w258 w264]
                  tunnel: w247 -> [w257 w263]
                  tunnel: w246 -> [_ w268]
                  tunnel: [w249 w267] -> w245
                  tunnel: [w250 w266] -> w244
                  frame False {
                    w256 = u16 0 items=["Decelerate", "Halt"] ("Motion Stop Type")
                    n57 = call <vilib>:"Single Axis Move Stop.vi"("error in (no error)"=w257, "Motion Stop Type"=w256, "Axis Select"=Axis_Select."Axis 1", "GECO Motion in"=w258) -> ("error out"=w253:errorcluster, "Axis Select out"=w252:T15, "GECO Motion out"=w254:refnum<class "GECO Motion.lvclass">)  [unwired: 5 in]
                    n58 = call <vilib>:"Single Axis Load Velocity Override.vi"("error in (no error)"=w253, "Override Velosity Value"=0, "Axis Select"=w252, "GECO Motion in"=w254) -> ("error out"=w250:errorcluster, "GECO Motion out"=w249:refnum<class "GECO Motion.lvclass">)  [unwired: 5 in, 1 out]
                  }
                  frame True {
                    w262 = u16 0 items=["Decelerate", "Halt"] ("Motion Stop Type")
                    n59 = call <vilib>:"Single Axis Move Stop.vi"("error in (no error)"=w263, "Motion Stop Type"=w262, "Axis Select"=Axis_Select."Axis 2", "GECO Motion in"=w264) -> ("error out"=w260:errorcluster, "Axis Select out"=w259:T15, "GECO Motion out"=w261:refnum<class "GECO Motion.lvclass">)  [unwired: 5 in]
                    n60 = call <vilib>:"Single Axis Move Start.vi"("error in (no error)"=w260, "Axis Select"=w259, "GECO Motion in"=w261) -> ("error out"=w270:errorcluster, "Axis Select out"=w269:T15, "GECO Motion out"=w271:refnum<class "GECO Motion.lvclass">)  [unwired: 6 in]
                    n61 = call <vilib>:"Single Axis Load Velocity Override.vi"("error in (no error)"=w270, "Override Velosity Value"=w268, "Axis Select"=w269, "GECO Motion in"=w271) -> ("error out"=w266:errorcluster, "GECO Motion out"=w267:refnum<class "GECO Motion.lvclass">)  [unwired: 5 in, 1 out]
                  }
                }
              }
              frame 3 {
                n62 = Unbundle By Name(w273) -> ("二軸後退"=w272:bool)
                n63 = case shown="True" w272 {
                  tunnel: w278 -> [w288 w292]
                  tunnel: w277 -> [w287 w291]
                  tunnel: w276 -> [_ w300]
                  tunnel: [w279 w299] -> w275
                  tunnel: [w280 w298] -> w274
                  frame False {
                    w286 = u16 0 items=["Decelerate", "Halt"] ("Motion Stop Type")
                    n64 = call <vilib>:"Single Axis Move Stop.vi"("error in (no error)"=w287, "Motion Stop Type"=w286, "Axis Select"=Axis_Select."Axis 1", "GECO Motion in"=w288) -> ("error out"=w283:errorcluster, "Axis Select out"=w282:T15, "GECO Motion out"=w284:refnum<class "GECO Motion.lvclass">)  [unwired: 5 in]
                    n65 = call <vilib>:"Single Axis Load Velocity Override.vi"("error in (no error)"=w283, "Override Velosity Value"=0, "Axis Select"=w282, "GECO Motion in"=w284) -> ("error out"=w280:errorcluster, "GECO Motion out"=w279:refnum<class "GECO Motion.lvclass">)  [unwired: 5 in, 1 out]
                  }
                  frame True {
                    w290 = u16 0 items=["Decelerate", "Halt"] ("Motion Stop Type")
                    n66 = Multiply(x=-1, y=w300) -> (x*y=w297:i32)
                    n67 = call <vilib>:"Single Axis Move Stop.vi"("error in (no error)"=w291, "Motion Stop Type"=w290, "Axis Select"=Axis_Select."Axis 2", "GECO Motion in"=w292) -> ("error out"=w294:errorcluster, "Axis Select out"=w289:T15, "GECO Motion out"=w295:refnum<class "GECO Motion.lvclass">)  [unwired: 5 in]
                    n68 = call <vilib>:"Single Axis Move Start.vi"("error in (no error)"=w294, "Axis Select"=w289, "GECO Motion in"=w295) -> ("error out"=w302:errorcluster, "Axis Select out"=w301:T15, "GECO Motion out"=w303:refnum<class "GECO Motion.lvclass">)  [unwired: 6 in]
                    n69 = call <vilib>:"Single Axis Load Velocity Override.vi"("error in (no error)"=w302, "Override Velosity Value"=w297, "Axis Select"=w301, "GECO Motion in"=w303) -> ("error out"=w298:errorcluster, "GECO Motion out"=w299:refnum<class "GECO Motion.lvclass">)  [unwired: 5 in, 1 out]
                  }
                }
              }
              frame 4 {
                n70 = Unbundle By Name(w305) -> ("三軸前進"=w304:bool)
                n71 = case shown="False" w304 {
                  tunnel: w310 -> [w320 w326]
                  tunnel: w309 -> [w319 w325]
                  tunnel: w308 -> [_ w330]
                  tunnel: [w311 w329] -> w307
                  tunnel: [w312 w328] -> w306
                  frame False {
                    w318 = u16 0 items=["Decelerate", "Halt"] ("Motion Stop Type")
                    n72 = call <vilib>:"Single Axis Move Stop.vi"("error in (no error)"=w319, "Motion Stop Type"=w318, "Axis Select"=Axis_Select."Axis 1", "GECO Motion in"=w320) -> ("error out"=w315:errorcluster, "Axis Select out"=w314:T15, "GECO Motion out"=w316:refnum<class "GECO Motion.lvclass">)  [unwired: 5 in]
                    n73 = call <vilib>:"Single Axis Load Velocity Override.vi"("error in (no error)"=w315, "Override Velosity Value"=0, "Axis Select"=w314, "GECO Motion in"=w316) -> ("error out"=w312:errorcluster, "GECO Motion out"=w311:refnum<class "GECO Motion.lvclass">)  [unwired: 5 in, 1 out]
                  }
                  frame True {
                    w324 = u16 0 items=["Decelerate", "Halt"] ("Motion Stop Type")
                    n74 = call <vilib>:"Single Axis Move Stop.vi"("error in (no error)"=w325, "Motion Stop Type"=w324, "Axis Select"=Axis_Select."Axis 3", "GECO Motion in"=w326) -> ("error out"=w322:errorcluster, "Axis Select out"=w321:T15, "GECO Motion out"=w323:refnum<class "GECO Motion.lvclass">)  [unwired: 5 in]
                    n75 = call <vilib>:"Single Axis Move Start.vi"("error in (no error)"=w322, "Axis Select"=w321, "GECO Motion in"=w323) -> ("error out"=w332:errorcluster, "Axis Select out"=w331:T15, "GECO Motion out"=w333:refnum<class "GECO Motion.lvclass">)  [unwired: 6 in]
                    n76 = call <vilib>:"Single Axis Load Velocity Override.vi"("error in (no error)"=w332, "Override Velosity Value"=w330, "Axis Select"=w331, "GECO Motion in"=w333) -> ("error out"=w328:errorcluster, "GECO Motion out"=w329:refnum<class "GECO Motion.lvclass">)  [unwired: 5 in, 1 out]
                  }
                }
              }
              frame 5 {
                n77 = Unbundle By Name(w335) -> ("三軸後退"=w334:bool)
                n78 = case shown="False" w334 {
                  tunnel: w340 -> [w350 w354]
                  tunnel: w339 -> [w349 w353]
                  tunnel: w338 -> [_ w362]
                  tunnel: [w341 w361] -> w337
                  tunnel: [w342 w360] -> w336
                  frame False {
                    w348 = u16 0 items=["Decelerate", "Halt"] ("Motion Stop Type")
                    n79 = call <vilib>:"Single Axis Move Stop.vi"("error in (no error)"=w349, "Motion Stop Type"=w348, "Axis Select"=Axis_Select."Axis 1", "GECO Motion in"=w350) -> ("error out"=w345:errorcluster, "Axis Select out"=w344:T15, "GECO Motion out"=w346:refnum<class "GECO Motion.lvclass">)  [unwired: 5 in]
                    n80 = call <vilib>:"Single Axis Load Velocity Override.vi"("error in (no error)"=w345, "Override Velosity Value"=0, "Axis Select"=w344, "GECO Motion in"=w346) -> ("error out"=w342:errorcluster, "GECO Motion out"=w341:refnum<class "GECO Motion.lvclass">)  [unwired: 5 in, 1 out]
                  }
                  frame True {
                    w352 = u16 0 items=["Decelerate", "Halt"] ("Motion Stop Type")
                    n81 = Multiply(x=-1, y=w362) -> (x*y=w359:i32)
                    n82 = call <vilib>:"Single Axis Move Stop.vi"("error in (no error)"=w353, "Motion Stop Type"=w352, "Axis Select"=Axis_Select."Axis 3", "GECO Motion in"=w354) -> ("error out"=w356:errorcluster, "Axis Select out"=w351:T15, "GECO Motion out"=w357:refnum<class "GECO Motion.lvclass">)  [unwired: 5 in]
                    n83 = call <vilib>:"Single Axis Move Start.vi"("error in (no error)"=w356, "Axis Select"=w351, "GECO Motion in"=w357) -> ("error out"=w364:errorcluster, "Axis Select out"=w363:T15, "GECO Motion out"=w365:refnum<class "GECO Motion.lvclass">)  [unwired: 6 in]
                    n84 = call <vilib>:"Single Axis Load Velocity Override.vi"("error in (no error)"=w364, "Override Velosity Value"=w359, "Axis Select"=w363, "GECO Motion in"=w365) -> ("error out"=w360:errorcluster, "GECO Motion out"=w361:refnum<class "GECO Motion.lvclass">)  [unwired: 5 in, 1 out]
                  }
                }
              }
              frame 6 {
                n85 = Unbundle By Name(w367) -> ("三軸同進"=w366:bool)
                n86 = case shown="False" w366 {
                  tunnel: w372 -> [w376 w394]
                  tunnel: w371 -> [w377 w393]
                  tunnel: w370 -> [_ w389]
                  tunnel: [w374 w402] -> w369
                  tunnel: [w373 w401] -> w368
                  frame False {
                    w375 = T15[] [enum."Axis 1", enum."Axis 2", enum."Axis 3"] items=["Axis 1", "Axis 2", "Axis 3", "Axis 4"] ("Start Axes Select")
                    n87 = for {
                      tunnel: w377 -> [w386]
                      tunnel: w376 -> [w385]
                      tunnel: w375 -> [w384] mode=indexing
                      tunnel: [w379] -> w374
                      tunnel: [w380] -> w373
                      w387 = u16 0 items=["Decelerate", "Halt"] ("Motion Stop Type")
                      n88 = call <vilib>:"Single Axis Move Stop.vi"("error in (no error)"=w386, "Motion Stop Type"=w387, "Axis Select"=w384, "GECO Motion in"=w385) -> ("error out"=w382:errorcluster, "Axis Select out"=w381:T15, "GECO Motion out"=w383:refnum<class "GECO Motion.lvclass">)  [unwired: 5 in]
                      n89 = call <vilib>:"Single Axis Load Velocity Override.vi"("error in (no error)"=w382, "Override Velosity Value"=0, "Axis Select"=w381, "GECO Motion in"=w383) -> ("error out"=w380:errorcluster, "GECO Motion out"=w379:refnum<class "GECO Motion.lvclass">)  [unwired: 5 in, 1 out]
                    }
                  }
                  frame True {
                    w390 = T15[] [enum."Axis 1", enum."Axis 2", enum."Axis 3"] items=["Axis 1", "Axis 2", "Axis 3", "Axis 4"] ("Start Axes Select")
                    n90 = call <vilib>:"Single Axis Load Velocity Override.vi"("error in (no error)"=w393, "Override Velosity Value"=w389, "Axis Select"=Axis_Select."Axis 1", "GECO Motion in"=w394) -> ("error out"=w399:errorcluster, "GECO Motion out"=w400:refnum<class "GECO Motion.lvclass">)  [unwired: 5 in, 1 out]
                    n91 = call <vilib>:"Single Axis Load Velocity Override.vi"("error in (no error)"=w399, "Override Velosity Value"=w389, "Axis Select"=Axis_Select."Axis 2", "GECO Motion in"=w400) -> ("error out"=w397:errorcluster, "GECO Motion out"=w398:refnum<class "GECO Motion.lvclass">)  [unwired: 5 in, 1 out]
                    n92 = call <vilib>:"Single Axis Load Velocity Override.vi"("error in (no error)"=w397, "Override Velosity Value"=w389, "Axis Select"=Axis_Select."Axis 3", "GECO Motion in"=w398) -> ("error out"=w395:errorcluster, "GECO Motion out"=w396:refnum<class "GECO Motion.lvclass">)  [unwired: 5 in, 1 out]
                    n93 = call <vilib>:"MultiAxes Sync Move Start.vi"("error in (no error)"=w395, "Start Axes Select"=w390, "GECO Motion in"=w396) -> ("error out"=w401:errorcluster, "GECO Motion out"=w402:refnum<class "GECO Motion.lvclass">)  [unwired: 7 in]
                  }
                }
              }
              frame 7 {
                n94 = Unbundle By Name(w404) -> ("三軸同退"=w403:bool)
                n95 = case shown="False" w403 {
                  tunnel: w409 -> [w413 w433]
                  tunnel: w408 -> [w414 w432]
                  tunnel: w407 -> [_ w426]
                  tunnel: [w411 w441] -> w406
                  tunnel: [w410 w440] -> w405
                  frame False {
                    w412 = T15[] [enum."Axis 1", enum."Axis 2", enum."Axis 3"] items=["Axis 1", "Axis 2", "Axis 3", "Axis 4"] ("Start Axes Select")
                    n96 = for {
                      tunnel: w414 -> [w423]
                      tunnel: w413 -> [w422]
                      tunnel: w412 -> [w421] mode=indexing
                      tunnel: [w416] -> w411
                      tunnel: [w417] -> w410
                      w424 = u16 0 items=["Decelerate", "Halt"] ("Motion Stop Type")
                      n97 = call <vilib>:"Single Axis Move Stop.vi"("error in (no error)"=w423, "Motion Stop Type"=w424, "Axis Select"=w421, "GECO Motion in"=w422) -> ("error out"=w419:errorcluster, "Axis Select out"=w418:T15, "GECO Motion out"=w420:refnum<class "GECO Motion.lvclass">)  [unwired: 5 in]
                      n98 = call <vilib>:"Single Axis Load Velocity Override.vi"("error in (no error)"=w419, "Override Velosity Value"=0, "Axis Select"=w418, "GECO Motion in"=w420) -> ("error out"=w417:errorcluster, "GECO Motion out"=w416:refnum<class "GECO Motion.lvclass">)  [unwired: 5 in, 1 out]
                    }
                  }
                  frame True {
                    w429 = T15[] [enum."Axis 1", enum."Axis 2", enum."Axis 3"] items=["Axis 1", "Axis 2", "Axis 3", "Axis 4"] ("Start Axes Select")
                    n99 = Multiply(x=w426, y=-1) -> (x*y=w427:i32)
                    n100 = call <vilib>:"Single Axis Load Velocity Override.vi"("error in (no error)"=w432, "Override Velosity Value"=w427, "Axis Select"=Axis_Select."Axis 1", "GECO Motion in"=w433) -> ("error out"=w438:errorcluster, "GECO Motion out"=w439:refnum<class "GECO Motion.lvclass">)  [unwired: 5 in, 1 out]
                    n101 = call <vilib>:"Single Axis Load Velocity Override.vi"("error in (no error)"=w438, "Override Velosity Value"=w427, "Axis Select"=Axis_Select."Axis 2", "GECO Motion in"=w439) -> ("error out"=w436:errorcluster, "GECO Motion out"=w437:refnum<class "GECO Motion.lvclass">)  [unwired: 5 in, 1 out]
                    n102 = call <vilib>:"Single Axis Load Velocity Override.vi"("error in (no error)"=w436, "Override Velosity Value"=w427, "Axis Select"=Axis_Select."Axis 3", "GECO Motion in"=w437) -> ("error out"=w434:errorcluster, "GECO Motion out"=w435:refnum<class "GECO Motion.lvclass">)  [unwired: 5 in, 1 out]
                    n103 = call <vilib>:"MultiAxes Sync Move Start.vi"("error in (no error)"=w434, "Start Axes Select"=w429, "GECO Motion in"=w435) -> ("error out"=w440:errorcluster, "GECO Motion out"=w441:refnum<class "GECO Motion.lvclass">)  [unwired: 7 in]
                  }
                }
              }
            }
            n104 = Bundle By Name(cluster=w156, "GECO Motion out"=w157) -> (w162:T14)
            n105 = Enqueue Element(queue=w154, element=T12 {"CMD"="PanelUpdate", "DATA"=variant}, error in (no error)=w155) -> (error out=w153:errorcluster)  [unwired: 1 in, 2 out]
          }
          frame "ZABMove" {
            w443 = T15[] [enum."Axis 1", enum."Axis 2", enum."Axis 3"] items=["Axis 1", "Axis 2", "Axis 3", "Axis 4"] ("Start Axes Select")
            n106 = Unbundle By Name(w455) -> ("PIDSetting.Move Setting"=w456:T20, "GECO Motion out"=w444:refnum<class "GECO Motion.lvclass">)
            n107 = call <vilib>:"MultiAxes Sync Move Start.vi"("error in (no error)"=w445, "Start Axes Select"=w443, "GECO Motion in"=w444) -> ("error out"=w446:errorcluster, "GECO Motion out"=w447:refnum<class "GECO Motion.lvclass">)  [unwired: 7 in]
            n108 = case shown="1" w456 {
              selector: w456 -> [_ w476 w586 _ _]
              tunnel: w455 -> [_ w498 w580 w601 w604]
              tunnel: w446 -> [w461 w507 w582 w600 w603]
              tunnel: [w460 w468 w531 w600 w603] -> w454
              tunnel: [w459 w477 w529 w599 w602] -> w452
              tunnel: w451 -> [_ w470 w530 _ _]
              tunnel: [_ _ w585 _ _] -> w450
              tunnel: [_ _ w584 _ _] -> w449
              tunnel: [_ _ w583 _ _] -> w448
              tunnel: w447 -> [w457 _ w581 _ _]
              tunnel: [_ _ w516 _ _] -> w442
              frame Default {
                w458 = T15[] [enum."Axis 1", enum."Axis 2", enum."Axis 3", enum."Axis 4"] items=["Axis 1", "Axis 2", "Axis 3", "Axis 4"]
                n109 = for {
                  tunnel: w461 -> [w464]
                  tunnel: [w462] -> w460
                  tunnel: [w463] -> w459
                  tunnel: w458 -> [w466] mode=indexing
                  tunnel: w457 -> [w467]
                  w465 = u16 0 items=["Decelerate", "Halt"] ("Motion Stop Type")
                  n110 = call <vilib>:"Single Axis Move Stop.vi"("error in (no error)"=w464, "Motion Stop Type"=w465, "Axis Select"=w466, "GECO Motion in"=w467) -> ("error out"=w462:errorcluster, "GECO Motion out"=w463:refnum<class "GECO Motion.lvclass">)  [unwired: 5 in, 1 out]
                }
              }
              frame 0 {
                w486 = T15[] [enum."Axis 1", enum."Axis 2", enum."Axis 3"] items=["Axis 1", "Axis 2", "Axis 3", "Axis 4"] ("Start Axes Select")
                # "輸入Z、A、B"
                n111 = Unbundle By Name(w498) -> ("PIDSetting.Z"=w504:i32, "PIDSetting.A"=w503:i32, "PIDSetting.B"=w502:i32, "PIDSetting.Axis Length"=w512:dbl, "PIDSetting.Axis Pulse"=w508:dbl, "GECO Motion out"=w506:refnum<class "GECO Motion.lvclass">)
                n112 = Unbundle By Name(w498) -> ("ServoSetting.Singel Axis Move Paramters.Velocity (10000)"=w481:i32)
                n113 = call "綜合圓軌跡子VI.vi"("Ring"=w476, "移動z"=w504, "al"=w503, "be"=w502) -> ("Z"=w478:dbl, "A"=w479:dbl, "B"=w480:dbl)  [unwired: 2 in]
                n114 = call "推導公式.vi"("be"=w480, "al"=w479, "移動z"=w478) -> ("L3"=w513:dbl, "L2"=w514:dbl, "L1"=w515:dbl)
                n115 = Subtract(x=w515, y=w512) -> (x-y=w511:dbl)
                n116 = Subtract(x=w514, y=w512) -> (x-y=w510:dbl)
                n117 = Subtract(x=w513, y=w512) -> (x-y=w509:dbl)
                n118 = Multiply(x=w511, y=w508) -> (x*y=w474:dbl)
                n119 = Multiply(x=w510, y=w508) -> (x*y=w483:dbl)
                n120 = Multiply(x=w509, y=w508) -> (x*y=w475:dbl)
                n121 = call <vilib>:"Single Axis Load Velocity Override.vi"("error in (no error)"=w507, "Override Velosity Value"=w481, "Axis Select"=Axis_Select."Axis 1" ("Single Axis Select"), "GECO Motion in"=w506) -> ("error out"=w500:errorcluster, "Axis Select out"=w499:T15, "GECO Motion out"=w501:refnum<class "GECO Motion.lvclass">)  [unwired: 5 in]
                n122 = call <vilib>:"Single Axis Load Position Override.vi"("error in (no error)"=w500, "Override Target Position Value"=w475, "Axis Select"=w499, "GECO Motion in"=w501) -> ("error out"=w496:errorcluster, "GECO Motion out"=w497:refnum<class "GECO Motion.lvclass">)  [unwired: 5 in, 1 out]
                n123 = call <vilib>:"Single Axis Load Velocity Override.vi"("error in (no error)"=w496, "Override Velosity Value"=w481, "Axis Select"=Axis_Select."Axis 2" ("Single Axis Select"), "GECO Motion in"=w497) -> ("error out"=w493:errorcluster, "Axis Select out"=w492:T15, "GECO Motion out"=w494:refnum<class "GECO Motion.lvclass">)  [unwired: 5 in]
                n124 = call <vilib>:"Single Axis Load Position Override.vi"("error in (no error)"=w493, "Override Target Position Value"=w483, "Axis Select"=w492, "GECO Motion in"=w494) -> ("error out"=w487:errorcluster, "GECO Motion out"=w488:refnum<class "GECO Motion.lvclass">)  [unwired: 5 in, 1 out]
                n125 = call <vilib>:"Single Axis Load Velocity Override.vi"("error in (no error)"=w487, "Override Velosity Value"=w481, "Axis Select"=Axis_Select."Axis 3" ("Single Axis Select"), "GECO Motion in"=w488) -> ("error out"=w490:errorcluster, "Axis Select out"=w489:T15, "GECO Motion out"=w491:refnum<class "GECO Motion.lvclass">)  [unwired: 5 in]
                n126 = call <vilib>:"Single Axis Load Position Override.vi"("error in (no error)"=w490, "Override Target Position Value"=w474, "Axis Select"=w489, "GECO Motion in"=w491) -> ("error out"=w484:errorcluster, "GECO Motion out"=w485:refnum<class "GECO Motion.lvclass">)  [unwired: 5 in, 1 out]
                n127 = call <vilib>:"MultiAxes Sync Move Start.vi"("error in (no error)"=w484, "Start Axes Select"=w486, "GECO Motion in"=w485) -> ("error out"=w469:errorcluster, "GECO Motion out"=w477:refnum<class "GECO Motion.lvclass">)  [unwired: 7 in]
                n128 = Flush Queue(queue=w470, error in (no error)=w469) -> (queue out=w473:refnum<queue>, error out=w472:errorcluster)  [unwired: 1 out]
                n129 = Enqueue Element(queue=w473, element=T12 {"CMD"="BoardAccess", "DATA"=variant}, error in (no error)=w472) -> (error out=w468:errorcluster)  [unwired: 1 in, 2 out]
              }
              frame 1 {
                w579 = cluster{"output high":dbl, "output low":dbl} {"output high"=200000.0, "output low"=-500000.0} ("PID Def Output range")
                w544 = Axis_Select."Axis 3" ("Single Axis Select")
                w545 = Axis_Select."Axis 2" ("Single Axis Select")
                w543 = Axis_Select."Axis 1" ("Single Axis Select")
                # "PID取樣時間"
                # "Stm32 Delay Time"
                # "圓軌跡"
                n130 = Unbundle By Name(w580) -> ("PIDSetting.Axis Length"=w552:dbl, "PIDSetting.Axis Pulse"=w569:dbl)
                n131 = feedback #1() -> (w520:i32)
                n132 = Increment(x=w520) -> (x+1=w521:i32)
                n133 = feedback-in #1(w521) -> ()
                n134 = call <vilib>:"Read Encoder Position.vi"("error in (no error)"=w582, "Axis Select"=w543, "GECO Motion in"=w581) -> ("error out"=w550:errorcluster, "GECO Motion out"=w551:refnum<class "GECO Motion.lvclass">, "Encoder Position"=w527:i32, "Logical Position"=w542:i32)  [unwired: 4 in, 1 out]
                n135 = call <vilib>:"Read Encoder Position.vi"("error in (no error)"=w550, "Axis Select"=w545, "GECO Motion in"=w551) -> ("error out"=w548:errorcluster, "GECO Motion out"=w549:refnum<class "GECO Motion.lvclass">, "Encoder Position"=w526:i32, "Logical Position"=w541:i32)  [unwired: 4 in, 1 out]
                n136 = Bundle("Encoder Position"=w527, "Logical Position"=w542) -> (w585:T1)  [unwired: 1 in]
                n137 = call <vilib>:"Read Encoder Position.vi"("error in (no error)"=w548, "Axis Select"=w544, "GECO Motion in"=w549) -> ("error out"=w546:errorcluster, "GECO Motion out"=w547:refnum<class "GECO Motion.lvclass">, "Encoder Position"=w525:i32, "Logical Position"=w540:i32)  [unwired: 4 in, 1 out]
                n138 = call "綜合圓軌跡子VI.vi"("Ring"=w586, "I時間"=w520) -> ("Z"=w576:dbl, "A"=w519:dbl, "B"=w518:dbl)  [unwired: 4 in]
                n139 = property on="Axis 1" class="Clust (strict)"("Value"=w585) -> ()  [unwired: 2 in, 2 out]
                n140 = call "推導公式.vi"("be"=w518, "al"=w519, "移動z"=w576) -> ("L3"=w570:dbl, "L2"=w571:dbl, "L1"=w572:dbl)
                n141 = Bundle("Encoder Position"=w526, "Logical Position"=w541) -> (w584:T1)  [unwired: 1 in]
                n142 = Subtract(x=w572, y=w552) -> (x-y=w575:dbl)
                n143 = Subtract(x=w571, y=w552) -> (x-y=w574:dbl)
                n144 = Subtract(x=w570, y=w552) -> (x-y=w573:dbl)
                n145 = property on="Axis 2" class="Clust (strict)"("Value"=w584) -> ()  [unwired: 2 in, 2 out]
                n146 = feedback #2() -> (w524:i32)
                n147 = feedback-in #2(w527) -> ()
                n148 = feedback #3() -> (w523:i32)
                n149 = feedback-in #3(w526) -> ()
                n150 = feedback #4() -> (w522:i32)
                n151 = feedback-in #4(w525) -> ()
                n152 = Multiply ("L1 pulse")(x=w575, y=w569) -> (x*y=w538:dbl)
                n153 = Multiply ("L2 pulse")(x=w574, y=w569) -> (x*y=w537:dbl)
                n154 = Multiply ("L3 pulse")(x=w573, y=w569) -> (x*y=w536:dbl)
                n155 = Divide(x=25.0, y=1000.0) -> (x/y=w565:dbl)
                n156 = Bundle("Encoder Position"=w525, "Logical Position"=w540) -> (w583:T1)  [unwired: 1 in]
                n157 = property on="Axis 3" class="Clust (strict)"("Value"=w583) -> ()  [unwired: 2 in, 2 out]
                n158 = call-poly <vilib>:"PID.vi"("output range"=w579, "dt (s)"=w565, "PID gains"="PID gains", "process variable"=w524, "setpoint"=w536) -> ("output"=w535:dbl)  [unwired: 5 in, 1 out]
                n159 = call-poly <vilib>:"PID.vi"("output range"=w579, "dt (s)"=w565, "PID gains"="PID gains 2", "process variable"=w523, "setpoint"=w537) -> ("output"=w534:dbl)  [unwired: 5 in, 1 out]
                n160 = call-poly <vilib>:"PID.vi"("output range"=w579, "dt (s)"=w565, "PID gains"="PID gains 3", "process variable"=w522, "setpoint"=w538) -> ("output"=w533:dbl)  [unwired: 5 in, 1 out]
                n161 = call <vilib>:"Single Axis Load Velocity Override.vi"("error in (no error)"=w546, "Override Velosity Value"=w535, "Axis Select"=w543, "GECO Motion in"=w547) -> ("error out"=w563:errorcluster, "Axis Select out"=w555:T15, "GECO Motion out"=w564:refnum<class "GECO Motion.lvclass">)  [unwired: 5 in]
                n162 = call <vilib>:"Single Axis Load Position Override.vi"("error in (no error)"=w563, "Axis Select"=w555, "GECO Motion in"=w564) -> ("error out"=w561:errorcluster, "GECO Motion out"=w562:refnum<class "GECO Motion.lvclass">)  [unwired: 6 in, 1 out]
                n163 = call <vilib>:"Single Axis Load Velocity Override.vi"("error in (no error)"=w561, "Override Velosity Value"=w534, "Axis Select"=w545, "GECO Motion in"=w562) -> ("error out"=w539:errorcluster, "Axis Select out"=w554:T15, "GECO Motion out"=w560:refnum<class "GECO Motion.lvclass">)  [unwired: 5 in]
                n164 = call <vilib>:"Single Axis Load Position Override.vi"("error in (no error)"=w539, "Axis Select"=w554, "GECO Motion in"=w560) -> ("error out"=w558:errorcluster, "GECO Motion out"=w559:refnum<class "GECO Motion.lvclass">)  [unwired: 6 in, 1 out]
                n165 = call <vilib>:"Single Axis Load Velocity Override.vi"("error in (no error)"=w558, "Override Velosity Value"=w533, "Axis Select"=w544, "GECO Motion in"=w559) -> ("error out"=w556:errorcluster, "Axis Select out"=w553:T15, "GECO Motion out"=w557:refnum<class "GECO Motion.lvclass">)  [unwired: 5 in]
                n166 = call <vilib>:"Single Axis Load Position Override.vi"("error in (no error)"=w556, "Axis Select"=w553, "GECO Motion in"=w557) -> ("error out"=w528:errorcluster, "GECO Motion out"=w529:refnum<class "GECO Motion.lvclass">)  [unwired: 6 in, 1 out]
                n167 = case shown="False" "ZABStop" {
                  tunnel: [w592 w595] -> w531
                  tunnel: w530 -> [w590 w594]
                  tunnel: w528 -> [w589 w593]
                  frame False {
                    n168 = Flush Queue(queue=w590, error in (no error)=w589) -> (queue out=w587:refnum<queue>, error out=w588:errorcluster)  [unwired: 1 out]
                    n169 = Enqueue Element(queue=w587, element=T12 {"CMD"="ZABMove", "DATA"=variant}, error in (no error)=w588) -> (error out=w592:errorcluster)  [unwired: 1 in, 2 out]
                  }
                  frame True {
                    n170 = Flush Queue(queue=w594, error in (no error)=w593) -> (queue out=w598:refnum<queue>, error out=w597:errorcluster)  [unwired: 1 out]
                    n171 = Enqueue Element(queue=w598, element=T12 {"CMD"="BoardAccess", "DATA"=variant}, error in (no error)=w597) -> (error out=w595:errorcluster)  [unwired: 1 in, 2 out]
                  }
                }
                n172 = Bundle By Name(cluster=cluster{"A":dbl, "B":dbl} {"A"=0.0, "B"=0.0} ("理想角度"), "A"=w519, "B"=w518) -> (w516:cluster{"A":dbl, "B":dbl})
              }
              frame 2 {
                # "Á³±Û­y¸ñ"
                n173 = Unbundle By Name(w601) -> ("GECO Motion out"=w599:refnum<class "GECO Motion.lvclass">)
              }
              frame 3 {
                # "Z上下"
                n174 = Unbundle By Name(w604) -> ("GECO Motion out"=w602:refnum<class "GECO Motion.lvclass">)
              }
            }
            n175 = Bundle By Name(cluster=w455, "GECO Motion out"=w452, "Axis 1 Position"=w450, "Axis 2 Position"=w449, "Axis 3 Position"=w448, "理想角度"=w442) -> (w453:T14)
          }
          frame "AlarmReset" {
            w611 = T15[] [enum."Axis 1", enum."Axis 2", enum."Axis 3", enum."Axis 4"] items=["Axis 1", "Axis 2", "Axis 3", "Axis 4"]
            n176 = Unbundle By Name(w610) -> ("GECO Motion out"=w608:refnum<class "GECO Motion.lvclass">)
            n177 = for {
              tunnel: [w620] -> w606
              tunnel: [w619] -> w605
              tunnel: w611 -> [w614] mode=indexing
              tunnel: w609 -> [w616]
              tunnel: w608 -> [w615]
              w612 = u16 0 items=["Decelerate", "Halt"] ("Motion Stop Type")
              n178 = call <vilib>:"Single Axis Move Stop.vi"("error in (no error)"=w616, "Motion Stop Type"=w612, "Axis Select"=w614, "GECO Motion in"=w615) -> ("error out"=w617:errorcluster, "Axis Select out"=w613:T15, "GECO Motion out"=w618:refnum<class "GECO Motion.lvclass">)  [unwired: 5 in]
              n179 = call <vilib>:"Alarm Reset.vi"("error in (no error)"=w617, "Axis Select"=w613, "GECO Motion in"=w618) -> ("error out"=w619:errorcluster, "GECO Motion out"=w620:refnum<class "GECO Motion.lvclass">)  [unwired: 6 in, 1 out]
            }
            n180 = Bundle By Name(cluster=w610, "GECO Motion out"=w606) -> (w607:T14)
          }
          frame "EncoderReset" {
            w627 = T15[] [enum."Axis 1", enum."Axis 2", enum."Axis 3", enum."Axis 4"] items=["Axis 1", "Axis 2", "Axis 3", "Axis 4"]
            n181 = Unbundle By Name(w626) -> ("GECO Motion out"=w624:refnum<class "GECO Motion.lvclass">)
            n182 = for {
              tunnel: [w636] -> w622
              tunnel: [w635] -> w621
              tunnel: w627 -> [w634] mode=indexing
              tunnel: w625 -> [w631]
              tunnel: w624 -> [w630]
              w628 = u16 0 items=["Decelerate", "Halt"] ("Motion Stop Type")
              n183 = call <vilib>:"Single Axis Move Stop.vi"("error in (no error)"=w631, "Motion Stop Type"=w628, "Axis Select"=w634, "GECO Motion in"=w630) -> ("error out"=w632:errorcluster, "Axis Select out"=w629:T15, "GECO Motion out"=w633:refnum<class "GECO Motion.lvclass">)  [unwired: 5 in]
              n184 = call <vilib>:"Reset Encoder Position.vi"("error in (no error)"=w632, "Axis Select"=w629, "GECO Motion in"=w633) -> ("error out"=w635:errorcluster, "GECO Motion out"=w636:refnum<class "GECO Motion.lvclass">)  [unwired: 6 in, 1 out]
            }
            n185 = Bundle By Name(cluster=w626, "GECO Motion out"=w622) -> (w623:T14)
          }
          frame "LinkBoard" {
            n186 = Unbundle By Name(w660) -> ("resource name"=w647:tag, "TCP slave port"=w658:u16, "ServoSetting.Motion Controller Slot"=w648:T18)
            n187 = Format Date/Time String(time format string (%c)="%Y %m %d %H %M ") -> (date/time string=w644:string)  [unwired: 2 in]
            n188 = Concatenate Strings(w644, "Ideal Angle.txt" ("element")) -> (w643:string)
            n189 = Build Path(base path=path "C:/Users/baby3/OneDrive/Desktop/碩論/陀螺儀監控平台控制/GyroData", name or relative path=w643) -> (appended path=w645:path)
            n190 = Open/Create/Replace File(file path (use dialog)=w645, error in=w639, operation (0:open)=T25."replace or create") -> (refnum out=w637:refnum<file>, error out=w640:errorcluster)  [unwired: 3 in, 1 out]
            n191 = call-poly <vilib>:"Create Modbus Instance.vi"("error in"=w640, "port (502)"=w658) -> ("error out"=w657:errorcluster, "TCP slave instance"=w649:refnum<class "Modbus Slave.lvclass">)  [unwired: 8 in]
            n192 = call-poly <vilib>:"Initialize.vi"("error in (no error)"=w657, "resource name"=w647) -> ("error out"=w653:errorcluster, "GECO_Driver out"=w650:refnum<class "GECO_Driver.lvclass">)  [unwired: 8 in]
            n193 = call <vilib>:"Initialize Motion Controller.vi"("error in (no error)"=w653, "Slot"=w648, "GECO_Driver in"=w650) -> ("error out"=w651:errorcluster, "Motion reference out"=w652:refnum<class "GECO Motion.lvclass">)  [unwired: 7 in]
            n194 = Bundle By Name(cluster=w660, "Modbus COM"=w649, "GECO_Driver out"=w650, "GECO Motion out"=w652, "Save Path"=w637) -> (w659:T14)
            n195 = Enqueue Element(queue=w654, element=T12 {"CMD"="BoardAccess", "DATA"=variant}, error in (no error)=w651) -> (error out=w656:errorcluster)  [unwired: 1 in, 2 out]
          }
          frame "BoardAccess" {
            n196 = Unbundle By Name(w674) -> ("Modbus COM"=w671:refnum<class "Modbus API.lvclass">, "address starting"=w670:u16, "number of inputs"=w669:u16)
            n197 = call-dynamic "Read Holding Registers.vi"("error in"=w667, "number of inputs"=w669, "starting address"=w670, "Modbus instance in"=w671) -> ("error out"=w661:errorcluster, "register values"=w672:u16[])  [unwired: 5 in, 1 out]
            n198 = Enqueue Element(queue=w668, element=T12 {"CMD"="PanelUpdate", "DATA"=variant}, error in (no error)=w661) -> (queue out=w666:refnum<queue>, error out=w665:errorcluster)  [unwired: 1 in, 1 out]
            n199 = Bundle By Name(cluster=w674, "register values"=w672) -> (w673:T14)
            n200 = Enqueue Element(queue=w666, element=T12 {"CMD"="BoardAccess", "DATA"=variant}, error in (no error)=w665) -> (error out=w664:errorcluster)  [unwired: 1 in, 2 out]
          }
          frame "PanelUpdate" {
            n201 = Unbundle By Name(w697) -> ("GECO Motion out"=w696:refnum<class "GECO Motion.lvclass">)
            n202 = call <vilib>:"Read Encoder Position.vi"("error in (no error)"=w699, "Axis Select"=Axis_Select."Axis 1", "GECO Motion in"=w696) -> ("error out"=w692:errorcluster, "GECO Motion out"=w693:refnum<class "GECO Motion.lvclass">, "Encoder Position"=w685:i32, "Logical Position"=w686:i32)  [unwired: 4 in, 1 out]
            n203 = Bundle(cluster=T26 {"Logical Position"=0, "Encoder Position"=0} ("input cluster"), "Logical Position"=w686, "Encoder Position"=w685) -> (w677:T26)
            "Axis 1" <- w677
            n204 = call <vilib>:"Read Encoder Position.vi"("error in (no error)"=w692, "Axis Select"=Axis_Select."Axis 2", "GECO Motion in"=w693) -> ("error out"=w690:errorcluster, "GECO Motion out"=w691:refnum<class "GECO Motion.lvclass">, "Encoder Position"=w678:i32, "Logical Position"=w679:i32)  [unwired: 4 in, 1 out]
            n205 = Bundle(cluster=T26 {"Logical Position"=0, "Encoder Position"=0} ("input cluster"), "Logical Position"=w679, "Encoder Position"=w678) -> (w676:T26)
            "Axis 2" <- w676
            n206 = Unbundle By Name(w697) -> ("register values"=→"register values":i16[])
            n207 = call <vilib>:"Read Encoder Position.vi"("error in (no error)"=w690, "Axis Select"=Axis_Select."Axis 3", "GECO Motion in"=w691) -> ("error out"=w698:errorcluster, "GECO Motion out"=w694:refnum<class "GECO Motion.lvclass">, "Encoder Position"=w680:i32, "Logical Position"=w681:i32)  [unwired: 4 in, 1 out]
            n208 = Bundle(cluster=T26 {"Logical Position"=0, "Encoder Position"=0} ("input cluster"), "Logical Position"=w681, "Encoder Position"=w680) -> (w675:T26)
            "Axis 3" <- w675
            n209 = Bundle By Name(cluster=w697, "GECO Motion out"=w694, "Axis 1 Position"=w677, "Axis 2 Position"=w676, "Axis 3 Position"=w675) -> (w695:T14)
          }
          frame "CloseBoard" {
            w701 = T15[] [enum."Axis 1", enum."Axis 2", enum."Axis 3", enum."Axis 4"] items=["Axis 1", "Axis 2", "Axis 3", "Axis 4"]
            n210 = Unbundle By Name(w709) -> ("GECO_Driver out"=w703:refnum<class "GECO_Driver.lvclass">, "GECO Motion out"=w702:refnum<class "GECO Motion.lvclass">)
            n211 = Flush Queue(queue=w707, error in (no error)=w706) -> (error out=w705:errorcluster)  [unwired: 2 out]
            n212 = for {
              tunnel: [w714] -> w704
              tunnel: w702 -> [w713]
              tunnel: w705 -> [w712]
              tunnel: w701 -> [w710] mode=indexing
              n213 = call <vilib>:"Servo On.vi"("error in (no error)"=w712, "Servo On"=FALSE, "Axis Select"=w710, "GECO Motion in"=w713) -> ("error out"=w717:errorcluster, "Axis Select out"=w716:T15, "GECO Motion out"=w715:refnum<class "GECO Motion.lvclass">)  [unwired: 5 in]
              n214 = call <vilib>:"Single Axis Move Stop.vi"("error in (no error)"=w717, "Axis Select"=w716, "GECO Motion in"=w715) -> ("error out"=w714:errorcluster)  [unwired: 6 in, 2 out]
            }
            n215 = call <vilib>:"Close.vi"("error in (no error)"=w704, "GECO_Driver in"=w703) -> ("error out"=w708:errorcluster)  [unwired: 9 in]
          }
        }
        n216 = Unbundle By Name(w49) -> ("status"=w50:bool)
      }
      frame Error {
      }
    }
    n217 = Tick Count (ms)() -> (millisecond timer value=w41:u32)
    n218 = Unbundle By Name(w39) -> ("理想角度"=w38:cluster{"A":dbl, "B":dbl})
    n219 = Subtract(x=w41, y=w40) -> (x-y=w37:u32)
    "Program Period" <- w37
  }
  "error IO" <- w2
  n220 = while {
    tunnel: w21 -> [w733]
    tunnel: w19 -> [w732]
    shift-right: [w727] -> w11
    shift-left: T13 {"Byte bits"=0, "baud rate"=0, "實際角度"={"A"=0.0, "B"=0.0}, "COM Port"="", "Save Path"=refnum} -> [w728]
    tunnel: [w726] -> w4 mode=indexing
    shift-right: [w725] -> _
    shift-left: _ -> [w724]
    tunnel: [w722] -> w1
    tunnel: [w721] -> w5 mode=indexing
    stop <- w723 stop-if-true
    # "Gyro"
    n221 = Dequeue Element(queue=w733, error in (no error)=w732) -> (queue out=w730:refnum<queue>, element=w729:T12, error out=w731:errorcluster)  [unwired: 1 in, 1 out]
    n222 = case shown="No Error" w731 {
      selector: w731 -> [w737 w789]
      tunnel: w730 -> [w736 _]
      tunnel: w729 -> [w741 _]
      tunnel: [w735 TRUE] -> w723
      tunnel: w728 -> [w739 w790]
      tunnel: [w738 w790] -> w727
      tunnel: [w734 w789] -> w722
      frame No Error {
        n223 = Unbundle(w741) -> ("CMD"=w740:string)  [unwired: 1 out]
        n224 = case shown="\"GyroBoardAccess\"" w740 {
          tunnel: [w743 w749 w754 w767 w782 w784] -> w738
          tunnel: w739 -> [w743 w750 w751 w777 w782 w784]
          tunnel: w737 -> [w742 w745 w757 _ w781 w788]
          tunnel: [w742 w745 w755 w773 w781 w785] -> w734
          tunnel: w736 -> [_ _ w764 w776 _ w786]
          frame Default {
          }
          frame "Idle" {
            # "圖表歸零"
            n225 = property on="實際角度Chart" class="WFChart (strict)"("History Data"=cluster{"X":dbl, "Y":dbl}[] []) -> ()  [unwired: 2 in, 2 out]
            n226 = Bundle By Name(cluster=w750, "COM Port"="Serial Port", "baud rate"="baud rate", "Byte bits"="Byte bits") -> (w749:T13)
          }
          frame "GyroLink" {
            n227 = Format Date/Time String(time format string (%c)="%Y %m %d %H %M ") -> (date/time string=w762:string)  [unwired: 2 in]
            n228 = Concatenate Strings(w762, "GYro Angle.txt" ("element")) -> (w759:string)
            n229 = Enqueue Element(queue=w764, element=T12 {"CMD"="GyroBoardAccess", "DATA"=variant}, error in (no error)=w757) -> (error out=w756:errorcluster)  [unwired: 1 in, 2 out]
            n230 = Build Path(base path=path "C:/Users/baby3/OneDrive/Desktop/碩論/陀螺儀監控平台控制/GyroData", name or relative path=w759) -> (appended path=w758:path)
            n231 = Open/Create/Replace File(file path (use dialog)=w758, error in=w756, operation (0:open)=T25."replace or create") -> (refnum out=w753:refnum<file>, error out=w755:errorcluster)  [unwired: 3 in, 1 out]
            n232 = Bundle By Name(cluster=w751, "Save Path"=w753) -> (w754:T13)
          }
          frame "GyroBoardAccess" {
            n233 = Unbundle By Name(w777) -> ("COM Port"=w770:refnum<visa-resource-name>)
            n234 = call-poly "VISA Configure Serial Port"("VISA resource name"=w770, "baud rate (9600)"=u32 115200, "data bits (8)"=u16 8) -> ("VISA resource name out"=w769:refnum<visa-resource-name>, "error out"=w768:errorcluster)  [unwired: 11 in]
            n235 = VISA Read(VISA resource name=w769, byte count=u32 13, error in (no error)=w768) -> (read buffer=w780:string, error out=w779:errorcluster)  [unwired: 2 out]
            n236 = call "Arduino角度.vi"("error in"=w779, "read buffer"=w780) -> ("error out"=w774:errorcluster, "Waveform Chart"=w766:cluster{dbl, dbl})  [unwired: 2 in]
            "實際角度" <- w766
            "實際角度Chart" <- w766
            n237 = Enqueue Element(queue=w776, element=T12 {"CMD"="GyroBoardAccess", "DATA"=variant}, error in (no error)=w774) -> (error out=w773:errorcluster)  [unwired: 1 in, 2 out]
            n238 = Bundle By Name(cluster=w777, "實際角度"=w766) -> (w767:T13)
          }
          frame "GyroPanelUpdate" {
            n239 = Unbundle By Name(w782) -> ()  [unwired: 1 out]
          }
          frame "CloseBoard" {
            n240 = Unbundle By Name(w784) -> ("COM Port"=w783:refnum<visa-resource-name>)
            n241 = Flush Queue(queue=w786, error in (no error)=w788) -> (error out=w787:errorcluster)  [unwired: 2 out]
            n242 = VISA Close(VISA resource name=w783, error in (no error)=w787) -> (error out=w785:errorcluster)
          }
        }
        n243 = Unbundle By Name(w734) -> ("status"=w735:bool)
      }
      frame Error {
      }
    }
    n244 = Unbundle By Name(w727) -> ("實際角度"=w726:cluster{"A":dbl, "B":dbl})
    n245 = Tick Count (ms)() -> (millisecond timer value=w725:u32)
    n246 = Subtract(x=w725, y=w724) -> (x-y=w721:u32)
    "Gyro\nPeriod" <- w721
  }
  "error IO 2" <- w1
  n247 = Enqueue Element(queue=w21, element=T12 {"CMD"="Idle", "DATA"=variant}, error in (no error)=w24) -> (error out=w23:errorcluster)  [unwired: 1 in, 2 out]
  n248 = shared-variable ".\\RTVariables.lvlib\\MainProgramQueue"() -> ()  [unwired: 1 in, 2 out]
  n249 = while {
    shift-right: [w794] -> w35
    shift-left: w23 -> [w797]
    tunnel: w22 -> [w798]
    tunnel: w21 -> [w792]
    stop <- w795 stop-if-true
    # "EventLoop"
    n250 = event shown="[11] Panel Close?" {
      selector: _ -> [_ _ _ _ _ _ _ _ _ _ _ _]
      dyn-events: _ -> [_ _ _ _ _ _ _ _ _ _ _ _]
      timeout: _ -> [_ _ _ _ _ _ _ _ _ _ _ _]
      tunnel: w798 -> [w802 w806 w810 w817 w821 w825 w831 w835 _ _ w853 w856]
      tunnel: w797 -> [w801 w805 w809 w816 w820 w824 w830 w834 w841 w847 w852 w858]
      tunnel: [w800 w804 w808 w813 w819 w823 w829 w833 w840 w846 w850 w855] -> w794
      tunnel: [_ _ _ _ _ _ _ _ _ _ _ w860] -> w796
      tunnel: w792 -> [_ _ _ w811 _ _ _ _ w838 w844 w848 w859]
      event "Modbus Number of Inputs", "Serial Port", "TCP slave port", "baud rate", "Byte bits", "Modbus Address Starting": Value Change {
        n251 = event-data() -> ()  [unwired: 1 in, 1 out]
        n252 = Enqueue Element(queue=w802, element=T12 {"CMD"="SettingChange", "DATA"=variant}, error in (no error)=w801) -> (error out=w800:errorcluster)  [unwired: 1 in, 2 out]
      }
      event "Forward Enable?", "Reverse Enable?", "Motion Operation Mode", "Target Position (0)", "Acceleration (100000)", "Velocity (10000)", "Deacceleration (100000)", "Servo on": Value Change {
        n253 = event-data() -> ()  [unwired: 1 in, 1 out]
        n254 = Enqueue Element(queue=w806, element=T12 {"CMD"="ServoSetting", "DATA"=variant}, error in (no error)=w805) -> (error out=w804:errorcluster)  [unwired: 1 in, 2 out]
      }
      event "Z", "A", "B", "PID gains", "PID gains 2", "PID gains 3": Value Change {
        n255 = event-data() -> ()  [unwired: 1 in, 2 out]
        n256 = Enqueue Element(queue=w810, element=T12 {"CMD"="PIDSetting", "DATA"=variant}, error in (no error)=w809) -> (error out=w808:errorcluster)  [unwired: 1 in, 2 out]
      }
      event "Connect": Value Change {
        n257 = event-data() -> ()  [unwired: 1 in, 1 out]
        n258 = Enqueue Element(queue=w817, element=T12 {"CMD"="LinkBoard", "DATA"=variant}, error in (no error)=w816) -> (error out=w814:errorcluster)  [unwired: 1 in, 2 out]
        n259 = Enqueue Element(queue=w811, element=T12 {"CMD"="GyroLink", "DATA"=variant}, error in (no error)=w814) -> (error out=w813:errorcluster)  [unwired: 1 in, 2 out]
      }
      event "ServoButtonControl.AlarmReset": Value Change {
        n260 = event-data() -> ()  [unwired: 1 in, 1 out]
        n261 = Enqueue Element(queue=w821, element=T12 {"CMD"="AlarmReset", "DATA"=variant}, error in (no error)=w820) -> (error out=w819:errorcluster)  [unwired: 1 in, 2 out]
      }
      event "ServoButtonControl.Reset Encoder Position": Value Change {
        n262 = event-data() -> ()  [unwired: 1 in, 1 out]
        n263 = Enqueue Element(queue=w825, element=T12 {"CMD"="EncoderReset", "DATA"=variant}, error in (no error)=w824) -> (error out=w823:errorcluster)  [unwired: 1 in, 2 out]
      }
      event "ServoButtonControl": Value Change {
        n264 = event-data() -> ()  [unwired: 1 in, 1 out]
        n265 = Bundle By Name(cluster=T12 {"CMD"="Shooting", "DATA"=variant} ("element"), "DATA"="ServoButtonControl") -> (w827:T12)
        n266 = Enqueue Element(queue=w831, element=w827, error in (no error)=w830) -> (error out=w829:errorcluster)  [unwired: 1 in, 2 out]
      }
      event "ZABStop", "ZAB Start": Value Change {
        n267 = event-data() -> ()  [unwired: 1 in, 2 out]
        n268 = Enqueue Element(queue=w835, element=T12 {"CMD"="ZABMove", "DATA"=variant}, error in (no error)=w834) -> (error out=w833:errorcluster)  [unwired: 1 in, 2 out]
      }
      event "TimerON": Value Change {
        n269 = event-data() -> ("NewVal"=w836:bool)  [unwired: 1 in]
        n270 = Bundle By Name(cluster=T12 {"CMD"="ChangeTimerState", "DATA"=variant} ("element"), "DATA"=w836) -> (w837:T12)
        n271 = Enqueue Element(queue=w838, element=w837, error in (no error)=w841) -> (error out=w840:errorcluster)  [unwired: 1 in, 2 out]
      }
      event "Timer(ms)": Value Change {
        n272 = event-data() -> ("NewVal"=w842:i32)  [unwired: 1 in]
        n273 = Bundle By Name(cluster=T12 {"CMD"="ChangeTimerCount", "DATA"=variant} ("element"), "DATA"=w842) -> (w843:T12)
        n274 = Enqueue Element(queue=w844, element=w843, error in (no error)=w847) -> (error out=w846:errorcluster)  [unwired: 1 in, 2 out]
      }
      event "Close": Value Change {
        w849 = T12 {"CMD"="CloseBoard", "DATA"=variant} ("element")
        n275 = event-data() -> ()  [unwired: 1 in, 1 out]
        n276 = Enqueue Element At Opposite End(queue=w853, element=w849, error in (no error)=w852) -> (error out=w851:errorcluster)  [unwired: 1 in, 2 out]
        n277 = Enqueue Element At Opposite End(queue=w848, element=w849, error in (no error)=w851) -> (error out=w850:errorcluster)  [unwired: 1 in, 2 out]
      }
      event Panel Close? {
        w854 = T12 {"CMD"="CloseBoard", "DATA"=variant} ("element")
        w860 = TRUE
        n278 = event-data() -> ()  [unwired: 1 in, 1 out]
        n279 = Enqueue Element At Opposite End(queue=w859, element=w854, error in (no error)=w858) -> (error out=w857:errorcluster)  [unwired: 1 in, 2 out]
        n280 = event-data("Discard?"=w860) -> ()  [unwired: 1 in, 1 out]
        n281 = Enqueue Element At Opposite End(queue=w856, element=w854, error in (no error)=w857) -> (error out=w855:errorcluster)  [unwired: 1 in, 2 out]
      }
    }
    n282 = Unbundle By Name(w794) -> ("status"=w793:bool)
    n283 = Or(x=w793, y=w796) -> (x .or. y?=w795:bool)
  }
  n284 = Release Queue(queue=w21, error in (no error)=w35) -> (error out=w25:errorcluster)  [unwired: 1 in, 2 out]
  n285 = Release Queue(queue=w22, error in (no error)=w25) -> ()  [unwired: 1 in, 3 out]
  n286 = Unbundle By Name(w11) -> ("Save Path"=w10:refnum<file>)
  n287 = Unbundle By Name(w13) -> ("Save Path"=w12:refnum<file>)
  n288 = for {
    tunnel: [w870] -> w3 mode=indexing
    tunnel: w4 -> [w869] mode=indexing
    tunnel: w5 -> [w866] mode=indexing
    n289 = Unbundle(w869) -> ("A"=w868:dbl, "B"=w867:dbl)
    n290 = Format Into String(w868) -> (resulting string=w863:string)  [unwired: 3 in, 1 out]
    n291 = Format Into String(w867) -> (resulting string=w862:string)  [unwired: 3 in, 1 out]
    n292 = Format Into String(w866) -> (resulting string=w865:string)  [unwired: 3 in, 1 out]
    n293 = Insert Into Array(array=string[] ["Gyro Period(ms)："], new element #1=w865, new element #2="A：", new element #3=w863, new element #4="B：", new element #5=w862) -> (w870:string[])  [unwired: 1 in]
  }
  n294 = for {
    tunnel: [w881] -> w14 mode=indexing
    tunnel: w16 -> [w880] mode=indexing
    tunnel: w15 -> [w877] mode=indexing
    n295 = Unbundle(w880) -> ("A"=w879:dbl, "B"=w878:dbl)
    n296 = Format Into String(w879) -> (resulting string=w874:string)  [unwired: 3 in, 1 out]
    n297 = Format Into String(w878) -> (resulting string=w872:string)  [unwired: 3 in, 1 out]
    n298 = Format Into String(w877) -> (resulting string=w876:string)  [unwired: 3 in, 1 out]
    n299 = Insert Into Array(array=string[] ["Program Period(ms)："], new element #1=w876, new element #2="A：", new element #3=w874, new element #4="B：", new element #5=w872) -> (w881:string[])  [unwired: 1 in]
  }
  n300 = for {
    shift-right: [w885] -> w8
    shift-left: w10 -> [w887]
    shift-right: [w886] -> w9
    shift-left: _ -> [w884]
    tunnel: w3 -> [w883] mode=indexing
    n301 = Array To Spreadsheet String(delimiter (Tab)="\t", array=w883, 3:"%f" ("format string")) -> (spreadsheet string=w888:string)
    n302 = Write to Text File(file (use dialog)=w887, text=w888, error in=w884) -> (refnum out=w885:refnum<file>, error out=w886:errorcluster)  [unwired: 1 in, 1 out]
  }
  n303 = for {
    tunnel: w14 -> [w893] mode=indexing
    shift-right: [w891] -> w6
    shift-left: w12 -> [w895]
    shift-right: [w892] -> w7
    shift-left: _ -> [w894]
    n304 = Array To Spreadsheet String(delimiter (Tab)="\t", array=w893, 3:"%f" ("format string")) -> (spreadsheet string=w896:string)
    n305 = Write to Text File(file (use dialog)=w895, text=w896, error in=w894) -> (refnum out=w891:refnum<file>, error out=w892:errorcluster)  [unwired: 1 in, 1 out]
  }
  n306 = Close File(refnum=w8, error in=w9) -> ()  [unwired: 2 out]
  n307 = Close File(refnum=w6, error in=w7) -> ()  [unwired: 2 out]
